vi "Module - Page Execute.vi"(11 "Stop":bool) -> ()   [LabVIEW 2020]
uses:
  Control/State - eFGV.ctl
  Control/Page - Execute State.ctl
  <vilib>/Utility/miscctls.llb/LVPointDoubleTypeDef.ctl
  Control/Section.ctl
  Control/Execute - Index of Elapse time.ctl
  Control/State - FGV.ctl
  <vilib>/Utility/NIReport.llb/NI_report.lvclass
  <vilib>/Utility/NIReport.llb/Report Type.ctl
  <vilib>/Utility/NIReport.llb/NI_ReportGenerationCore.lvlib
  Control/Setup - Sequence Data.ctl
  Control/Transaction Info.ctl
  Control/Product Info.ctl
  Control/Acceptance Criteria Info.ctl
  Control/Execution Info.ctl
  Control/Results Info.ctl
  Control/Data to Execute.ctl
  <vilib>/Utility/file.llb/Write Delimited Spreadsheet (string).vi
  <userlib>/_OpenG.lib/comparison/comparison.llb/Boolean Changed__ogtk.vi
  Control/Drop Rate Param.ctl
  Control/Control 1.ctl
  <vilib>/Utility/NIReport.llb/Append Report Text (str wrap).vi
  Control/Setup - Sequence Data Label.ctl
panel:
  out "String.Stabilizing status":string
  in  "End Mark":bool caption="1"
  out "Test Status Ind":string="Testing"
  out "SequenceNoFolder":string="SeqNo2"
  out "Hold Time Remainder":dbl=833.0095882415771
  in  "TARE":bool caption="1"
  in  "Test Type":string(combo)
  in  "Execute Tab":enum32{"Test", "Info", "Misc."}(tab)
  in  "Chart No":string
  in  "View":string(combo)="Polar Plot"
  in  "Test Category":string
  in  "TabControl.TestType":enum32{"Holding", "Blowdown"}(tab)
  out "%Pressure Stabilized":dbl caption="% of Current Pressure on Top of\nThe Test Pressure" format="%.1f"
  out "% Test Completed":dbl format="%.1f"
  out "Holding Started":bool
  out "Bool. Press Drop In Range":bool caption="Drop Rate Within Range"
  out "Pressure in Range":bool
  out "NumInd.BD_Pressure":sgl caption="Blowdown pressure (psi)" format="%.1f"
  out "Bool.BDTrig":bool caption="Blowdown Triggered"
  out "NumInd.2nd_pump_press":sgl caption="Second pump pressure (psi)" format="%.1f"
  out "Overall Status":bool
  in  "Table Reading":i32(listbox)
  out "Low Pressure":bool
  in  "Pause/Resume":bool
  in  "Execute View":string="View"
  in  "Execute Reading":string="Reading"
  in  "Execute Key Value":string="Key Value" caption="Info"
  in  "Execute Info":string="Info" caption="Info"
  out "Blow Down  Test":bool
  out "Hold Time (hh:mm)":string="00:15"
  out "Test Pressure":i32=15000 format="%.0f psi"
  in  "tab - View Data":T1(tab)
  in  "Start Marker":u32(colorbox)=16860
  in  "Plot Colour":u32(colorbox)=16711680
  in  "Stop Marker":u32(colorbox)=1441830
  in  "Grid Colour":u32(colorbox)=35170
  out "Polar Plot":picture
  out "Linear Graph":cluster{"Time ,x":dbl[], "Magnitude ,y":sgl[]}(graph)={"Time ,x"=[0.0, 0.9682250022888184, 1.9675369262695312, 2.9678306579589844, 3.9680562019348145, 4.9682745933532715, 5.967533111572266, 6.9688215255737305, 7.969114303588867, 8.969351291656494, 9.968575954437256, 10.968814373016357, 11.96904182434082, 12.96934986114502, 13.968584060668945, 14.968928813934326, 15.970189094543457, 16.969515323638916, 17.969897747039795, 18.970128059387207, 19.971360206604004, 20.97115707397461, 21.97089910507202, 22.971266269683838, 23.970398426055908, 24.970824718475342, 25.97111749649048, 26.97133207321167, 27.970609664916992, 28.97120952606201, 29.971484184265137, 30.971708297729492, 31.971967220306396, 32.97223615646362, 33.97146987915039, 34.97170972824097, 35.972264766693115, 36.9714994430542, 37.9732346534729, 38.97247362136841, 39.973758697509766, 40.973976135253906, 41.97420263290405, 42.97359752655029, 43.973846435546875, 44.97406625747681, 45.9743447303772, 46.97364091873169, 47.97390556335449, 48.9737114906311, 49.97393465042114, 50.973427295684814, 51.97372102737427, 52.974024295806885, 53.97428226470947, 54.97451066970825, 55.974753856658936, 56.975521087646484, 57.97573757171631, 58.97601938247681, 59.977320194244385, 60.97653150558472, 61.97792720794678, 62.97848987579346, 63.9788384437561, 64.97906398773193, 65.97934484481812, 66.97858905792236, 67.97981309890747, 68.98035621643066, 69.97958898544312, 70.98087692260742, 71.98110103607178, 72.98132658004761, 73.98166465759277, 74.98196268081665, 75.98217439651489, 76.98144865036011, 77.98171186447144, 78.98278427124023, 79.98302412033081, 80.98324394226074, 81.98297834396362, 82.98421907424927, 83.98345279693604], "Magnitude ,y"=[15033.86, 15033.86, 15033.86, 15033.86, 15033.86, 15033.86, 15033.86, 15033.86, 15033.86, 15033.86, 15033.86, 15033.86, 15033.86, 6252.822, 6252.822, 6252.822, 6252.822, 15011.287, 15011.287, 15011.287, 15011.287, 15011.287, 15011.287, 15011.287, 15011.287, 15011.287, 15011.287, 15011.287, 15011.287, 15011.287, 15011.287, 15011.287, 15011.287, 15011.287, 15011.287, 15011.287, 15011.287, 15011.287, 15011.287, 15011.287, 15011.287, 15011.287, 15011.287, 15011.287, 15011.287, 15011.287, 15011.287, 15011.287, 15011.287, 15011.287, 15011.287, 15011.287, 15011.287, 15011.287, 15011.287, 15011.287, 15011.287, 15011.287, 15011.287, 15011.287, 15011.287, 15011.287, 15011.287, 15011.287, 15011.287, 15011.287, 15011.287, 15011.287, 15011.287, 15011.287, 15011.287, 15011.287, 15011.287, 15011.287, 15011.287, 15011.287, 15011.287, 15011.287, 15011.287, 15011.287, 15011.287, 15011.287, 15011.287, 15011.287, 15011.287]}
  in  "Statistic":i32(listbox)
  out "Key Value Remain Hold Time":string="00:00:00" caption="Holding Time Duration"
  out "Key Value Recording Duration":string="00:01:24" caption="Recording Duration"
  out "Key Value Current Pressure (psi)":sgl=15011.287 caption="Current Pressure (psi)"
  in  "Start Test":bool caption="1"
  out "Remaining Hold Time":string="00:00:00"
  out "Holding Pressure (psi)":dbl=15000.0
  out "Current Pressure (psi)":sgl
  in  "Clear Mark":bool caption="1"
  in  "Start Mark":bool caption="1"
  in  "Finish":bool caption="1"
  out "Start Holding Datetime":string="22.June.2022 06:14:10"
  out "Recorded Holding Time":string="00:03:00"
  out "Start Holding Pressure (psi)":string="15011.3"
  out "Different in Holding Pressure,psi(%)":string="0.0 psi(0.0 %)"
  out "Permitted Holding Pressure Drop, psi%":string="450.0 psi(3.0 %)"
  out "Recording Duration":string="00:00:00"
  out "Test Sequence":string="5"
  out "Seq.No":string="2"
  out "Variance":string="All"
  out "Transaction Number":u16=3
  out "Test Requirement":string="Hydro Open Body Test"
  out "Test Media":string="Water"
  out "Indicator.PressureDropRatePsi":dbl caption="Pressure Drop Rate" format="%.1f psi/hr"
  out "Indicator.PressureDropRate%":dbl caption="Pressure Drop Rate(psi/hr)" format="%.1f %%"
  out "Notes":string
  out "PSL":string
  in  "Test System Description":string caption="Test System"
  out "Rework":bool caption="Rework?"
  out "Ref Order No.":dbl caption="Ref. Order No."
  out "NCR No.":string
  in  "Header multi-test 3":T2={"Seq.Done"="Status", "Label.RunSeq"="Select", "Label.TestSeq"="Run?", "Label.SeqNo"="Test Sequence", "Seq.No 4"="Test Req. ID", "Seq.No 5"="Test Requirement", "Seq.No 6"="Variance", "Seq.No 7"="Test Procedure", "Seq.No 8"="Section", "Seq.No 9"="Test Bunker", "Seq.No 10"="Test Media", "Seq.No 11"="Test Pressure (psi)", "Seq.No 12"="Cycle", "Seq.No 13"="Holding time (hh:mm)", "Seq.No 14"="Chart Scale", "Seq.No 15"="Blowdown? (y/n)", "Seq.No 16"="Actuator Pressure (psi)", "Seq.No 17"="Max. Blowdown Pressure (psi)", "Label.SelectSeq"="No.", "Bool.SelectSeq"=FALSE, "Bool.RunSeq"=FALSE, "Bool.TestSeq"=FALSE, "Bool.SeqNo"=FALSE, "Label.TestGroup"="Test Group", "Bool.TestGroup"=FALSE, "Seq.MSHP"="MSHP", "Seq.PHPD"="PHPD"}
  out "Sequence List":T3[](array[typedef])=[{"Seq.Select"=FALSE, "Seq.Status"=6618880, "Seq.Run"=TRUE, "Seq.TestSequence"="5", "Seq.No"="1", "Seq.ReqID"="", "Seq.TestReq"="Hydro Open Body Test", "Seq.Variance"="All", "Seq.TestProcedure"="X-???", "Seq.Section"="???", "Seq.TestBunker"="SB SUT 1", "Seq.TestMedia"="Water", "Seq.TestPressure"="15000", "Seq.Cycle"="Primary", "Seq.HoldingTime"="00:03", "Seq.ChartScale"="", "Seq.BDIndicator"="N", "Seq.ActuatorPressure"="", "Seq.MaxBDPressure"=""}, {"Seq.Select"=FALSE, "Seq.Status"=3381759, "Seq.Run"=TRUE, "Seq.TestSequence"="5", "Seq.No"="2", "Seq.ReqID"="", "Seq.TestReq"="Hydro Open Body Test", "Seq.Variance"="All", "Seq.TestProcedure"="X-???", "Seq.Section"="???", "Seq.TestBunker"="SB SUT 1", "Seq.TestMedia"="Water", "Seq.TestPressure"="15000", "Seq.Cycle"="Secondary", "Seq.HoldingTime"="00:15", "Seq.ChartScale"="", "Seq.BDIndicator"="N", "Seq.ActuatorPressure"="", "Seq.MaxBDPressure"=""}, {"Seq.Select"=FALSE, "Seq.Status"=16711680, "Seq.Run"=TRUE, "Seq.TestSequence"="6", "Seq.No"="3", "Seq.ReqID"="", "Seq.TestReq"="Hydraulic Actuator/Bonnet Interface (PMV)", "Seq.Variance"="PMV", "Seq.TestProcedure"="X-341926-01", "Seq.Section"="???", "Seq.TestBunker"="SB SUT 1", "Seq.TestMedia"="Control Fluid", "Seq.TestPressure"="100", "Seq.Cycle"="Single Cycle", "Seq.HoldingTime"="00:03", "Seq.ChartScale"="", "Seq.BDIndicator"="N", "Seq.ActuatorPressure"="", "Seq.MaxBDPressure"=""}, {"Seq.Select"=FALSE, "Seq.Status"=16711680, "Seq.Run"=TRUE, "Seq.TestSequence"="6", "Seq.No"="4", "Seq.ReqID"="", "Seq.TestReq"="Hydraulic Actuator/Bonnet Interface (AMV)", "Seq.Variance"="AMV", "Seq.TestProcedure"="X-341926-01", "Seq.Section"="???", "Seq.TestBunker"="SB SUT 1", "Seq.TestMedia"="Control Fluid", "Seq.TestPressure"="100", "Seq.Cycle"="Single Cycle", "Seq.HoldingTime"="00:03", "Seq.ChartScale"="", "Seq.BDIndicator"="N", "Seq.ActuatorPressure"="", "Seq.MaxBDPressure"=""}]
  in  "Label.Test":string="Test" caption="Test"
  out "Test Category list":string="SUT 9, Hydro"
  in  "Test System":string
  in  "Test Category":string
  out "Material Description":string caption="Material List"
  out "Material":string="0"
  out "Project":string
  out "Customer Description":string caption="Customer List"
  in  "Test System Name":string
  in  "Procedure No./Ref.":string="X2345.xlsx" caption="X-Document No./Ref."
  out "Working Pressure":string
  in  "Test System":string
  out "Rev.":string
  out "Product Category":string
  out "BOM Rev.":dbl
  out "Sale Order":string="0" caption="Sales Order"
  out "Customer":string="0"
  out "NCR":string
  out "Order Number":string="0"
  out "Quantity":u16=1 min=1 step=1
  in  "Default View":string(combo)="Polar Plot"
  in  "View Change Duration":dbl=1.0 caption="Return to default view after" min=0.1 max=60.0 step=0.1 format="%.1f minutes"
  in  "Label.View change":string="Production Order Details" caption="Production Order Details"
  out "Enum.Pressure stabilize wait time":enum16{"seconds", "minutes"}(ring)=enum."minutes"
  out "Pressure stabilize wait time":dbl=10.0 min=0.0 max=100.0
  out "Auto Stop Test":bool caption="Automatic Stop Test after Hold Time Countdown"
  out "Auto Set Marker":bool=TRUE caption="Automatic set start marker upon pressure stabilized"
  in  "Header.Tool":T4={"Type "="Type", "Id"=" ID", "Description"="Description", "Serial No"="Serial No"} caption="Header Tool"
  out "Table.Tool":i32(listbox) caption="Detail Sensor"
  out "Table.Sensor":i32(listbox) caption="Detail Sensor"
  in  "Header.Sensor":T5={"Type "="Type", "Id"=" ID", "Description"="Description", "Serial No"="Serial No", "LP"="LP"} caption="Header Detail Sensor"
  in  "Label.Result":string="Result" caption="Result"
  out "Output Set Company":string
  out "ListBox.Output Set":string="1001.xltx" caption="Output Set"
  in  "Label.Production Order Details":string="Production Order Details" caption="Production Order Details"
  out "Indicator.Sub Operation":string caption="Sub Operation"
  out "Indicator.Confirmation No":u32 caption="Confirmation No"
  out "Indicator.Operation":string caption="Operation"
  out "Indicator.Sequence No":u16 caption="Sequence No"
  out "Indicator.Order Number":u32 caption="Order Number"
  in  "Label.Tools":string="Tools" caption="Tools"
  in  "Label.Sensor":string="Sensor" caption="Sensor"
  in  "Label.Additional Procedures No./Ref.":string="Additional Procedures No./Ref." caption="Additional Procedures No./Ref."
  out "Table.Procedure No./Ref.":i32(listbox)
  out "Acceptance Criteria":string="Acceptance Criteria"
  out "% Permitted Holding Pressure":string="% per hour (vs. start holding pressure)"
  out "% Test Pressure":string="% on top of the test pressure"
  out "Permitted Holding Pressure Drop":dbl=3.0
  out "Max Start Holding Pressure":dbl=3.0 caption="Maximum Start Of Holding Pressure"
  # "EXECUTE"
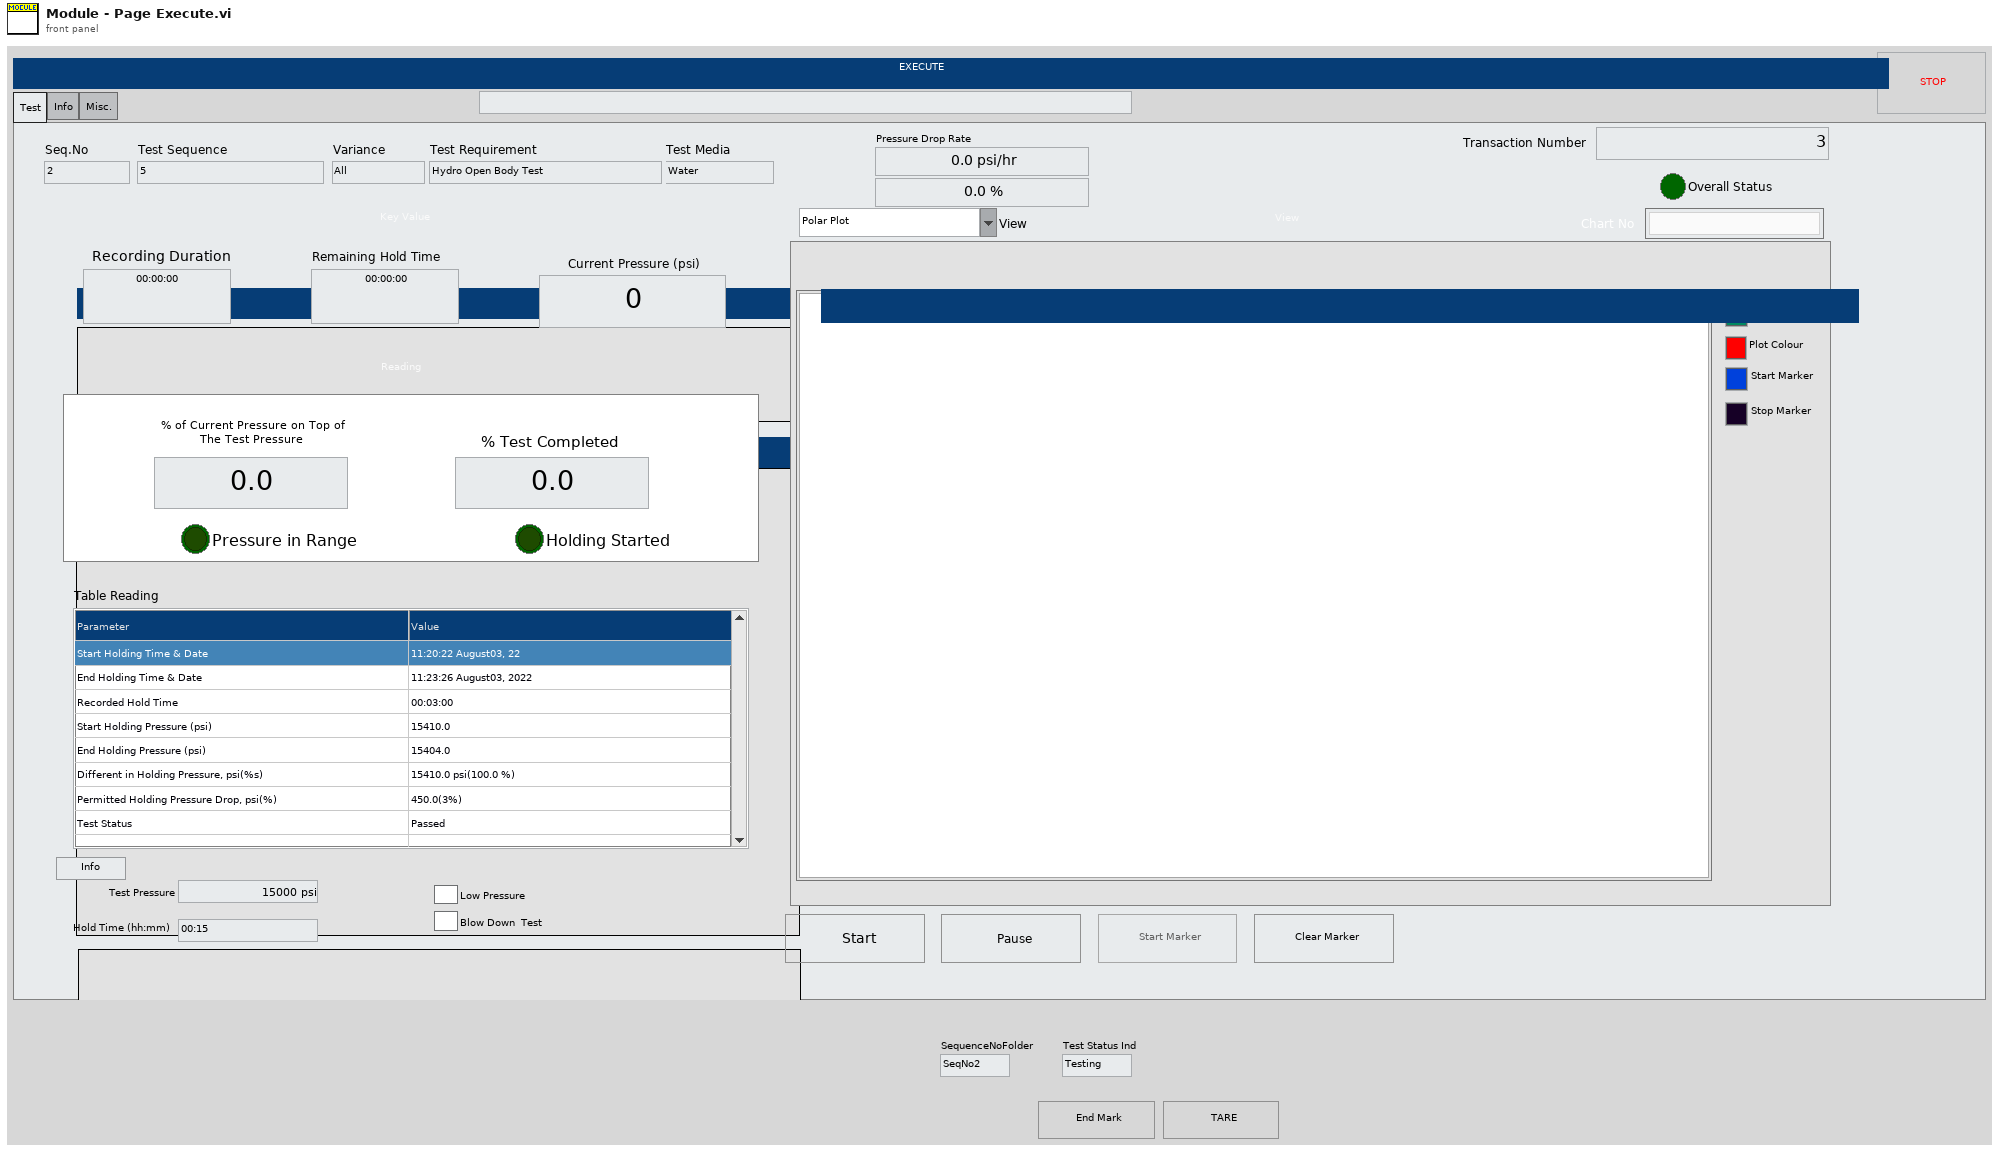
[diagram p1: front panel]
types:
  T1 = enum32{"Polar Plot", "Linear", "Statistic", "Key Value"}
  T2 = typedef "Setup - Sequence Data Label.ctl" = cluster{"Seq.Done":string, "Label.RunSeq":string, "Label.TestSeq":string, "Label.SeqNo":string, "Seq.No 4":string, "Seq.No 5":string, "Seq.No 6":string, "Seq.No 7":string, "Seq.No 8":string, "Seq.No 9":string, "Seq.No 10":string, "Seq.No 11":string, "Seq.No 12":string, "Seq.No 13":string, "Seq.No 14":string, "Seq.No 15":string, "Seq.No 16":string, "Seq.No 17":string, "Label.SelectSeq":string, "Bool.SelectSeq":bool, "Bool.RunSeq":bool, "Bool.TestSeq":bool, "Bool.SeqNo":bool, "Label.TestGroup":string, "Bool.TestGroup":bool, "Seq.MSHP":string, "Seq.PHPD":string}
  T3 = typedef "Setup - Sequence Data.ctl" = cluster{"Seq.Select":bool, "Seq.Status":u32, "Seq.Run":bool, "Seq.TestSequence":string, "Seq.No":string, "Seq.ReqID":string, "Seq.TestReq":string, "Seq.Variance":string, "Seq.TestProcedure":string, "Seq.Section":string, "Seq.TestBunker":string, "Seq.TestMedia":string, "Seq.TestPressure":string, "Seq.Cycle":string, "Seq.HoldingTime":string, "Seq.ChartScale":string, "Seq.BDIndicator":string, "Seq.ActuatorPressure":string, "Seq.MaxBDPressure":string}
  T4 = cluster{"Type ":string, "Id":string, "Description":string, "Serial No":string}
  T5 = cluster{"Type ":string, "Id":string, "Description":string, "Serial No":string, "LP":string}
  T6 = typedef "Execute - Index of Elapse time.ctl" = enum16{"Elapse Gap Data", "Holding Time", "Recording Duration", "View Change", "Pressure stabilize timer", "Press. Drop Rate", "Init Holding Buffer"}
  T7 = typedef "Data to Execute.ctl" = cluster{"Transaction Info":T8, "Product Info":T9, "Misc - Additional Refs":string[][], "Misc - Sensors":string[][], "Misc - Tools":string[][], "Acceptance Criteria Info":T10, "Execution Info":T11, "Results Info":T12, "Notes":string}
  T8 = typedef "Transaction Info.ctl" = cluster{"Transaction Number":string, "Order Number":string, "Quantity":u16, "Customer":u32, "Customer Description":string, "Project":string, "Sales Order":u32, "Material":string, "Material Description":string, "Rework":bool, "NCR No.":string, "Ref Order No.":string, "Item No.":u32, "BOM Rev.":dbl}
  T9 = typedef "Product Info.ctl" = cluster{"Product Category":string, "Procedure No./Ref.":string, "Test System":string, "Test System Description":string, "Working Pressure":string, "Pressure Unit":string, "Rev.":string, "PSL":string}
  T10 = typedef "Acceptance Criteria Info.ctl" = cluster{"Max Start Hold Pressure":dbl, "Enum.Max Start Hold Pressure":enum16{"%", "psi"}, "Permitted Hold Pressure Drop":dbl, "Enum.Permitted Hold Pressure Drop":enum16{"%", "psi"}, "Pressure stabilize wait time":dbl, "Enum.Pressure stabilize wait time":enum16{"seconds", "minutes"}}
  T11 = typedef "Execution Info.ctl" = cluster{"Auto Set Marker":bool, "Auto Stop Test":bool}
  T12 = typedef "Results Info.ctl" = cluster{"ListBox.Output Set":string, "Output Set Description":string}
  T13 = typedef "Setup - Sequence Data.ctl" = cluster{"Seq.Select":bool, "Seq.Status":u32, "Seq.Run":bool, "Seq.TestSequence":dbl, "Seq.No":dbl, "Seq.ReqID":string, "Seq.TestReq":string, "Seq.Variance":string, "Seq.TestProcedure":string, "Seq.Section":string, "Seq.TestSystem":string, "Seq.TestPressure":string, "Seq.Cycle":string, "Seq.TestGroup":dbl, "Seq.MSHP":dbl, "Seq.PHPD":dbl, "Seq.HoldingTime":string, "Seq.ChartScale":string, "Seq.ActuatorPressure":string, "Seq.MaxBDPressure":string, "Seq.BDIndicator":bool, "Seq.TestMedia":string}
  T14 = typedef "Drop Rate Param.ctl" = cluster{"Drop Rate Calc Interval (sec)":dbl, "Last Pressure (psi)":dbl, "Allowable Press. Drop/min":dbl, "Pressure Drop Accepted?":bool, "Block interval to test":i32, "Block counter":i32, "Allowable Press. Drop/hr":dbl}
  T15 = typedef "Control 1.ctl" = enum32{"Holding", "Blowdown"}
  T16 = cluster{"T_Out":i32, "Point Phase":dbl[], "polar attributes":cluster{"maximum":dbl, "minimum":dbl, "clip to min":bool, "log?(F)":bool, "grid color":u32, "plot color":u32, "fmt and prec":cluster{"format":enum8{"Decimal", "Scientific", "Engineering", "Binary", "Octal", "Hex"}, "precision":u8}, "visible section":u16}, "Current Pressure":sgl, "Counter Time":dbl, "marking plot colour":u32, "Active Cursor":u32, "Event AI Data":sgl[], "Run Test":bool, "Config":cluster{"Holding Pressure":dbl, "Set Polar Time":dbl}, "Array of Elapse Time":timestamp[], "Remaining Holding Time":dbl, "Max Pressure":sgl, "Start Mark":bool, "Plot length (min)":dbl, "Plot length scale":dbl, "Magnitude ,y":sgl[], "Time ,x":dbl[], "Result Elapse":dbl[], "Phase":dbl[], "data array [mag, phase (deg)]":cluster{"magnitude":dbl, "phase":dbl}[], "Max Phase":dbl, "Plot and scale":cluster{"Size Linear plot":u16, "Size point plot":u16, "Plot Scale":dbl}, "Start Holding Pressure (psi)":dbl, "End Holding Pressure (psi)":dbl, "Marking Data":cluster{"magnitude 2":dbl, "phase":dbl}[], "Display Polar Scale":cluster{"Time Scale Label":string, "Max Scale label":string}, "report out":refnum<class "NI_report.lvclass">, "axis labels":string[], "Polar Picture":picture, "Event Ref":refnum<event-registration>, "Data to Execute":T7, "Sequence Data":T13[], "Holding Started?":bool, "%Pressure Stabilized":dbl, "Target Holding Time":dbl, "Datalog path":path, "AI Offset":sgl[], "Sequence Number":i32, "Current Sequence":T13, "All Sequence Done":bool, "Sequence Started":bool, "Default View":string, "View Change Duration":dbl, "First data point?":bool, "Test Pressure Range":cluster{"Maximum":dbl, "Minimum":dbl, "Pressure in range?":bool}, "Stabilizing wait time":dbl, "Run Pressure Data":cluster{"Max Pressure":dbl, "Min Pressure":dbl, "Max Pressure TS":timestamp, "Min Pressure TS":timestamp}, "Drop Rate Param":T14, "TestType":T15, "Blowdown Param":cluster{"Actuator Pressure":dbl, "Max BD Pressure":dbl, "BD Triggered":bool, "BD Pressure":dbl}}
  T17 = typedef "Page - Execute State.ctl" = enum16{"Init", "Register Event", "Read Config File", "Idle", "Start Marking", "Clear Mark", "Init Test Param", "Init File and Folder", "Get Current Sequence", "Get pressure range", "Holding - Cal Elapse Time", "Get Current Pressure", "Calc. press. drop rate", "Check pressure in range", "Calc. stabilizing elapsed time", "Calc - Holding start Buffer Time", "Calc. Max Min Pressure", "Display Data", "Check Start Holding", "Blowdown - Check BD Trigger", "Blowdown - Mark BD", "Polar attributes", "Insert Acc Data", "Convert Time To Phase", "Get Plot length", "Polar linear Plot", "Polar Point", "Plot linear Graph", "Update Table Data", "Display Holding Time", "Display Result Test", "Display Label", "Finish Test", "Setup Cop", "Merge Picture", "Save  Data", "Get Next Sequence", "Create Report", "Fillup Report", "Process", "Update Info - Transaction", "Update Info - Product", "Update Info - Additional Refs", "Update Info - Sensors", "Update Info - Tools", "Update Info - Acceptance Criteria", "Update Info - Execution", "Update Info - Results", "Update Info - Notes", "Close"}
  T18 = typedef "Section.ctl" = enum16{"Software Setup", "Config", "Setup", "Network Stream", "MQTT Client", "Setting", "Sample Interval", "Calibration", "Pre-Ranging", "Overrun", "Static", "Filter", "Properties", "Alarm", "Device", "Logging"}
  T19 = typedef "LVPointDoubleTypeDef.ctl" = cluster{"X":dbl, "Y":dbl}
  T20 = typedef "State - FGV.ctl" = enum16{"Write", "Read"}
  T21 = enum8{"Decimal", "Scientific", "Engineering", "Binary", "Octal", "Hex"}
  T22 = cluster{"polar attributes":cluster{"maximum":dbl, "minimum":dbl, "clip to min":bool, "log?(F)":bool, "grid color":u32, "plot color":u32, "fmt and prec":cluster{"format":enum8{"Decimal", "Scientific", "Engineering", "Binary", "Octal", "Hex"}, "precision":u8}, "visible section":u16}, "data array [mag, phase (deg)]":cluster{"magnitude":dbl, "phase":dbl}[], "font":cluster{"desired font(Application) ":enum16{"User-specified Font", "Application Font", "System Font", "Dialog Font"}, "[user-specified font] ":cluster{"Font Name:":string, "Size":i16, "Strikeout?":bool, "Italic?":bool, "Underline?":bool, "Outline?":bool, "Shadow?":bool, "Bold?":bool}}, "Scale Polar plot":dbl, "Size":u16}
  T23 = cluster{"Execute Data":string[], "Sequence no":string}
  T24 = typedef "State - eFGV.ctl" = enum16{"Init", "Read", "Write", "Exit"}
  T25 = typedef "NI_ReportGenerationCore.lvlib/Report Type.ctl" = enum16{"HTML", "Word", "Excel"}
  T26 = cluster{"position (excel)":cluster{"row":i32, "column":i32}, "name (excel)":string, "bookmark (word)":string}
  T27 = enum8{"Enabled", "Disabled", "Disabled and Grayed Out"}
  T28 = cluster{"Maximum":dbl, "Minimum":dbl, "Pressure in range?":bool}
  T29 = cluster{"Size Linear plot":u16, "Size point plot":u16, "Plot Scale":dbl}
  T30 = cluster{"maximum":dbl, "minimum":dbl, "clip to min":bool, "log?(F)":bool, "grid color":u32, "plot color":u32, "fmt and prec":cluster{"format":enum8{"Decimal", "Scientific", "Engineering", "Binary", "Octal", "Hex"}, "precision":u8}, "visible section":u16}
  T31 = typedef "LVBoundsTypeDef.ctl" = cluster{"Width":u32, "Height":u32}
  T32 = typedef "imagedata.ctl" = cluster{"image type":i32, "image depth":i32, "image":u8[], "mask":u8[], "colors":u32[], "Rectangle":cluster{"left":i16, "top":i16, "right":i16, "bottom":i16}}
  T33 = enum32{"invalid app kind", "Development System", "Run Time System", "Student Edition", "Embedded LabVIEW", "Evaluation", "Custom"}
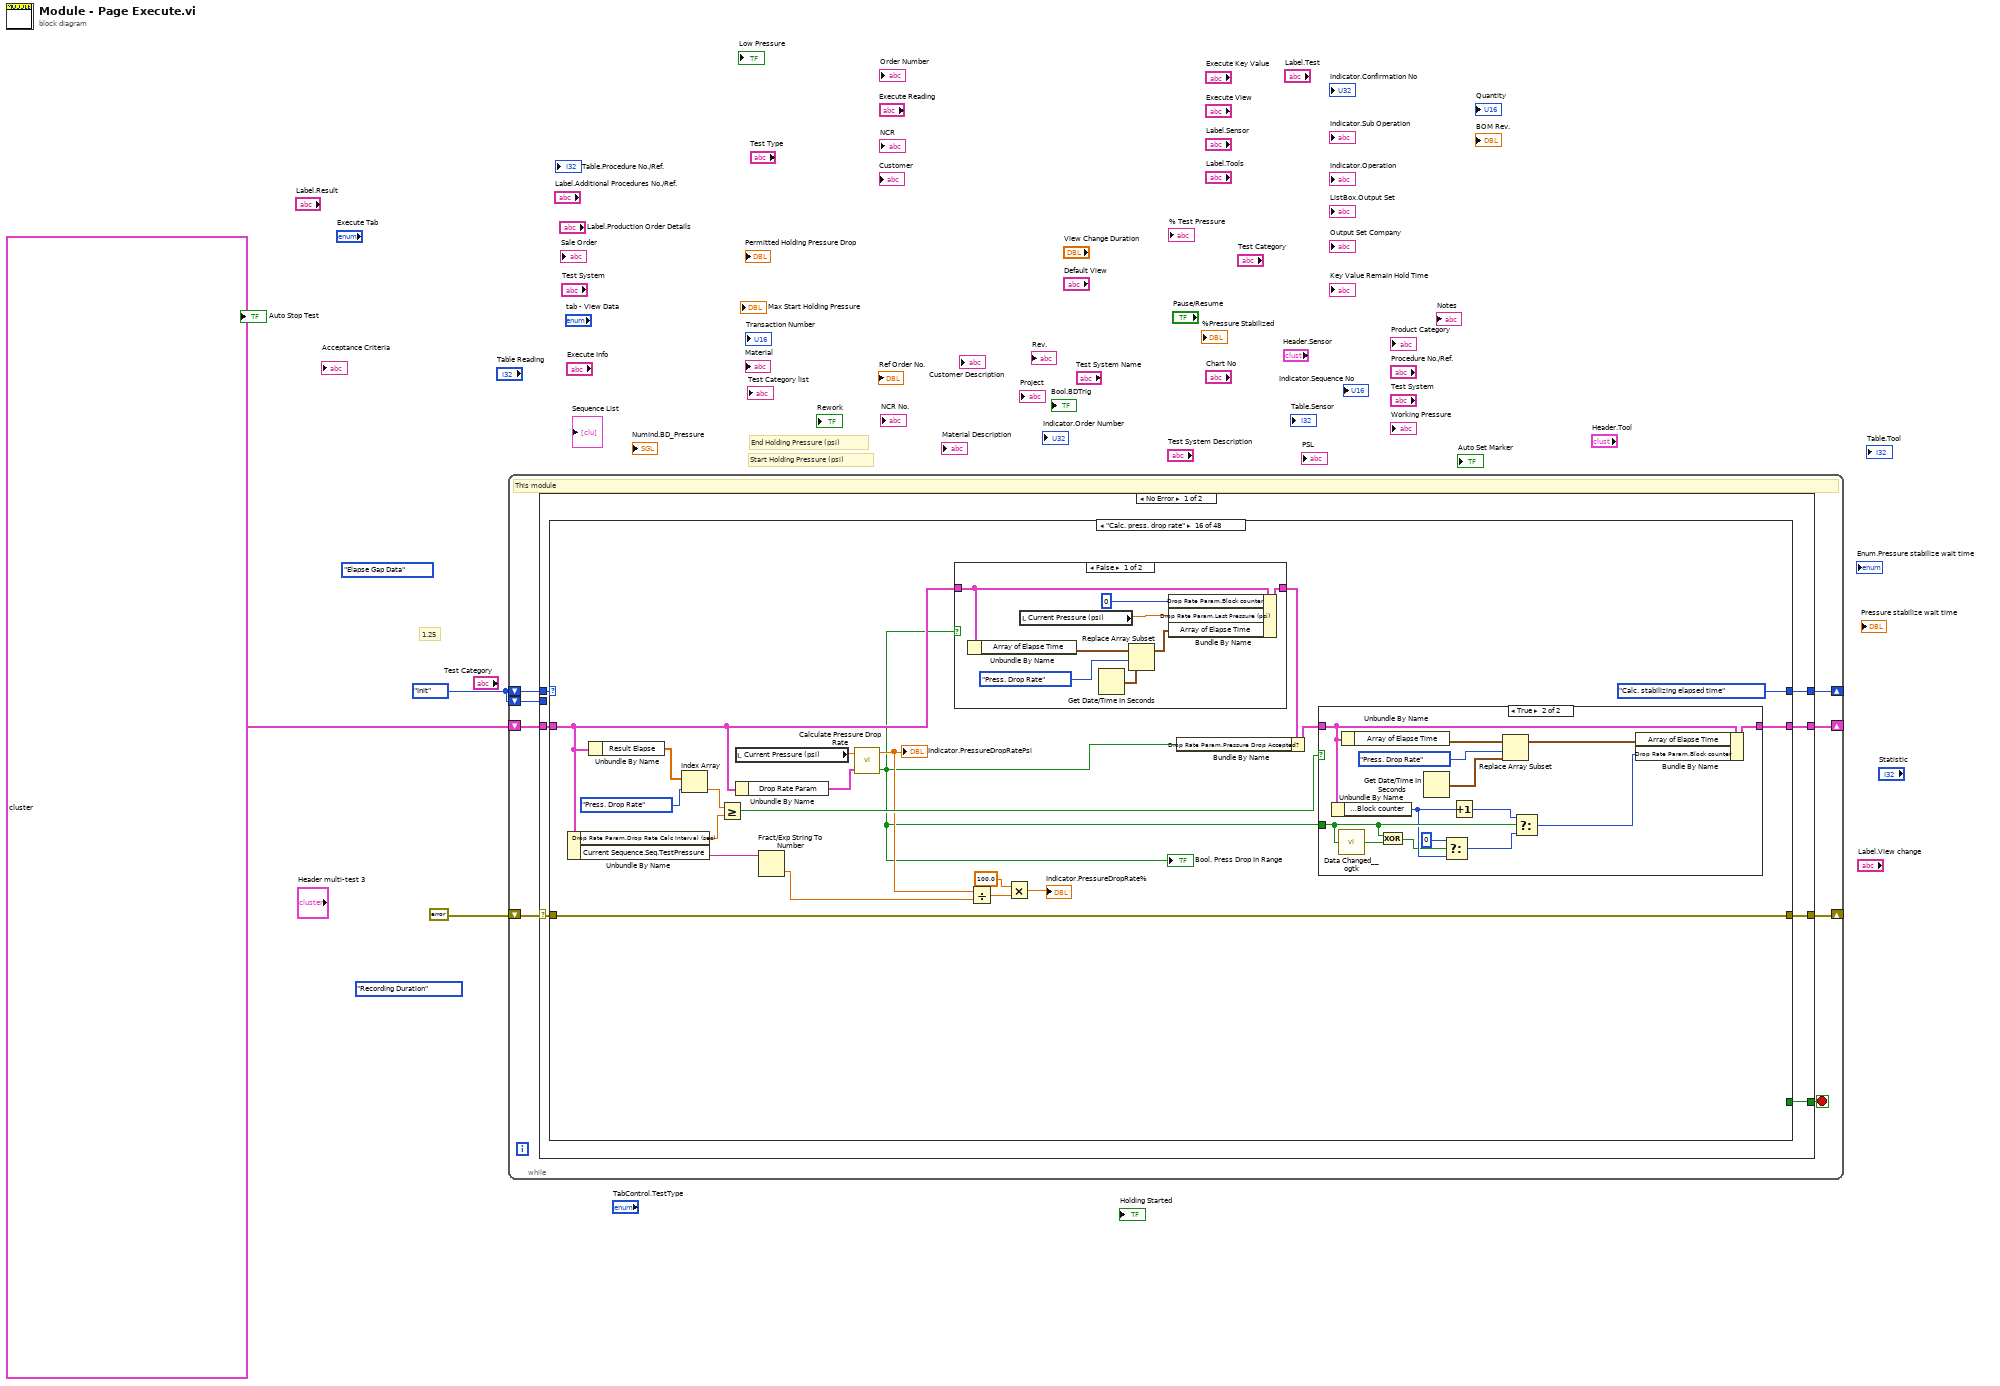
[diagram p0: block diagram]
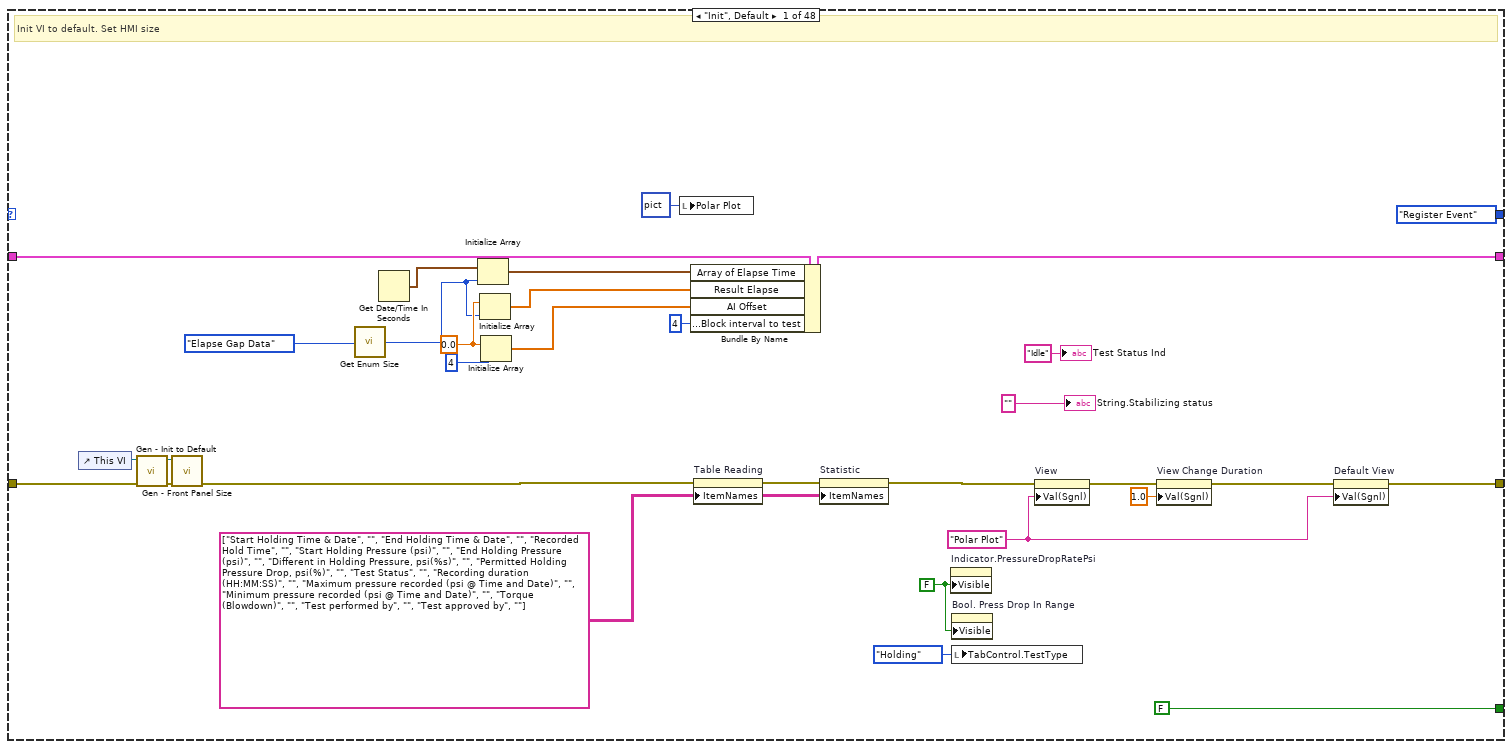
[diagram p2: hidden frame]
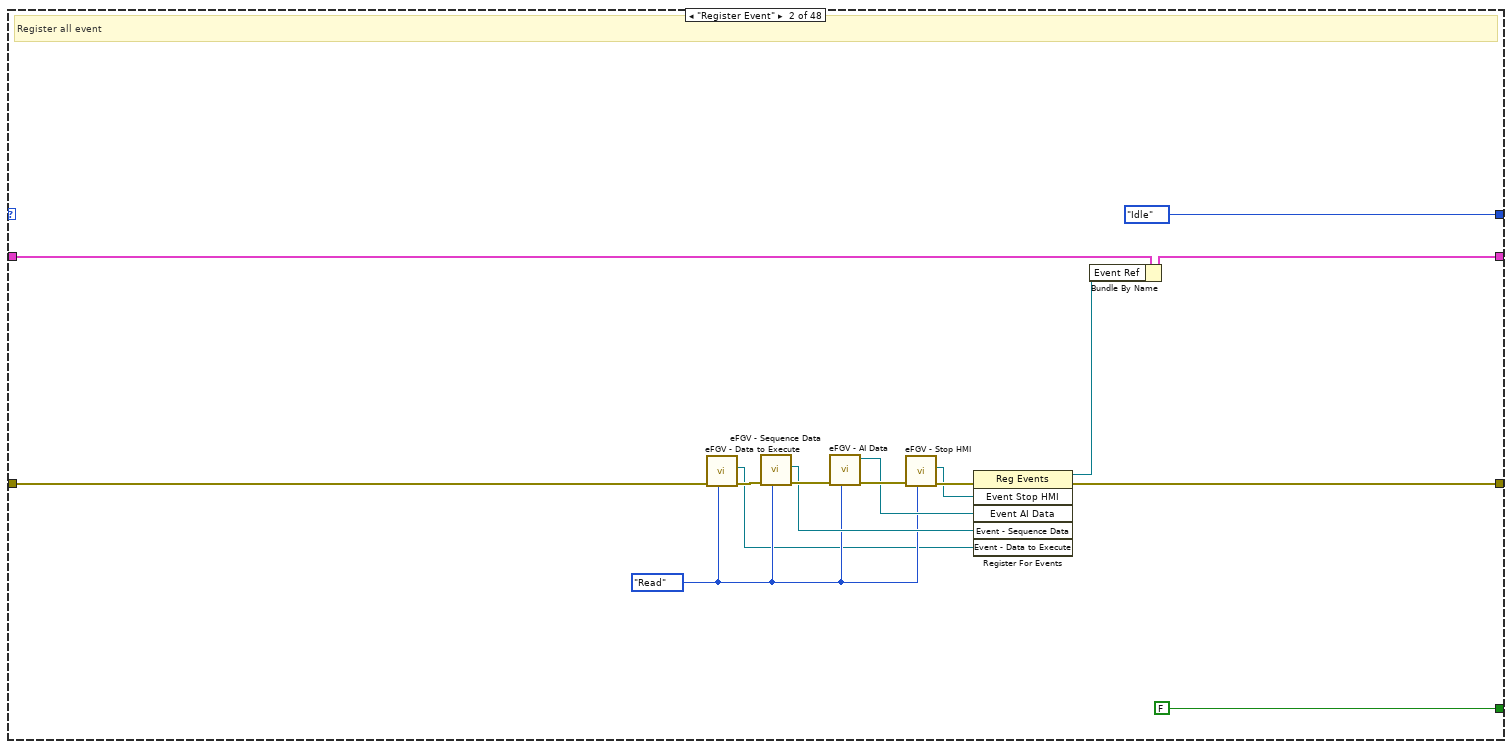
[diagram p3: hidden frame]
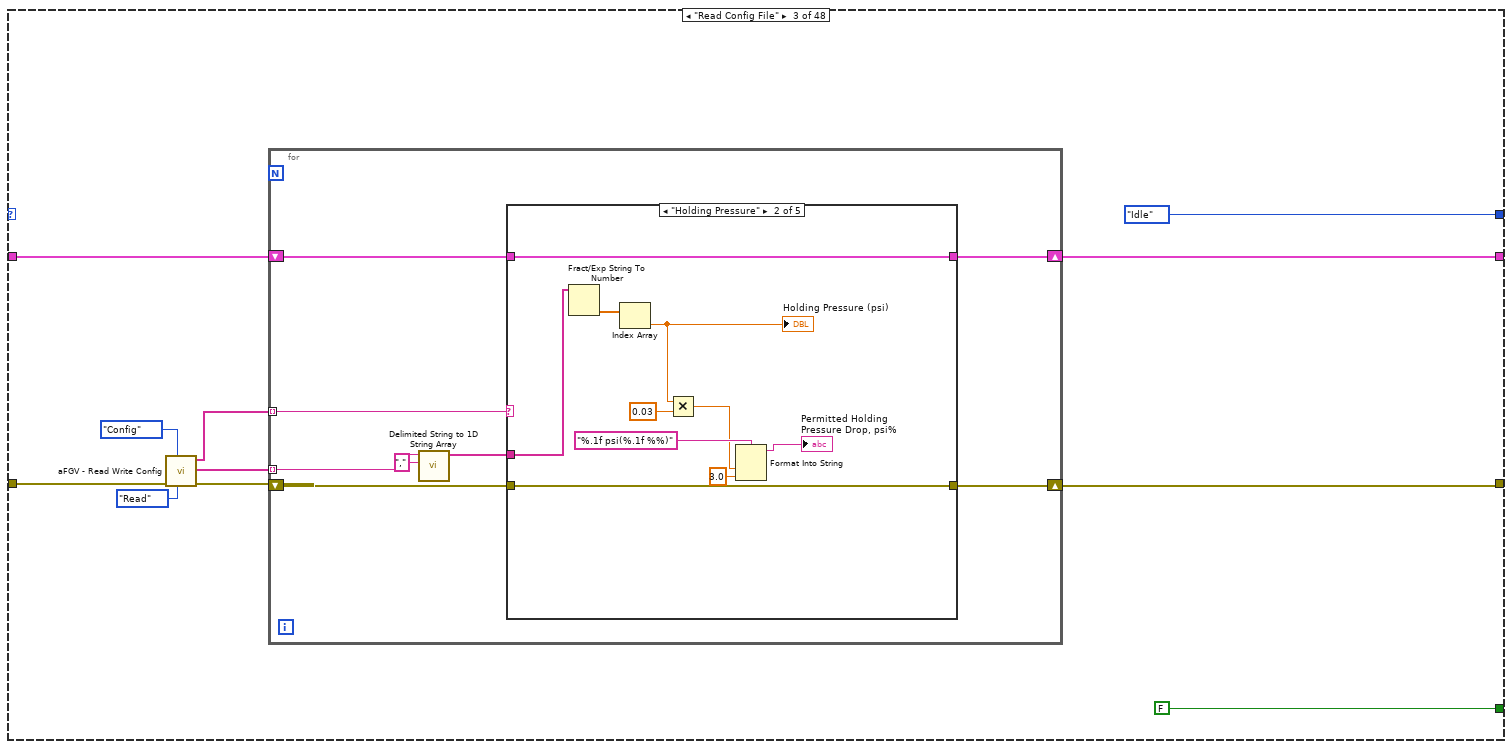
[diagram p4: hidden frame]
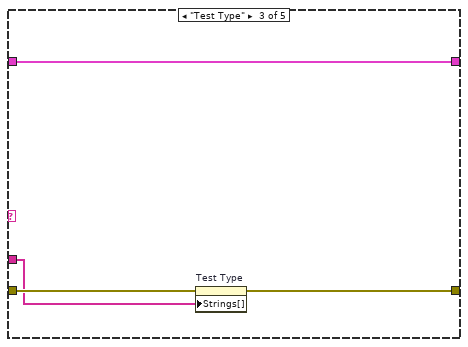
[diagram p6: hidden frame]
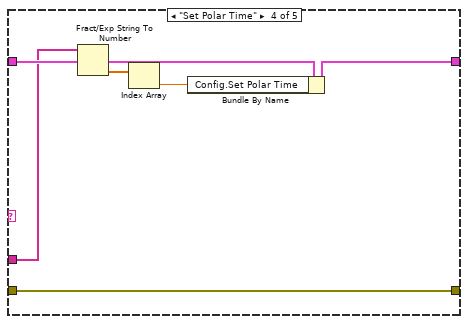
[diagram p7: hidden frame]
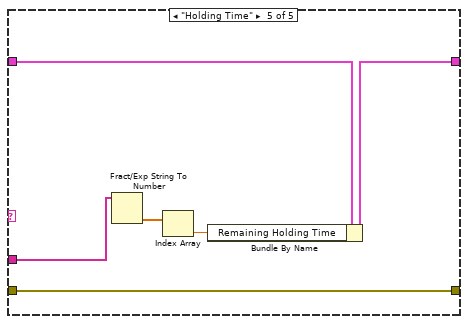
[diagram p8: hidden frame]
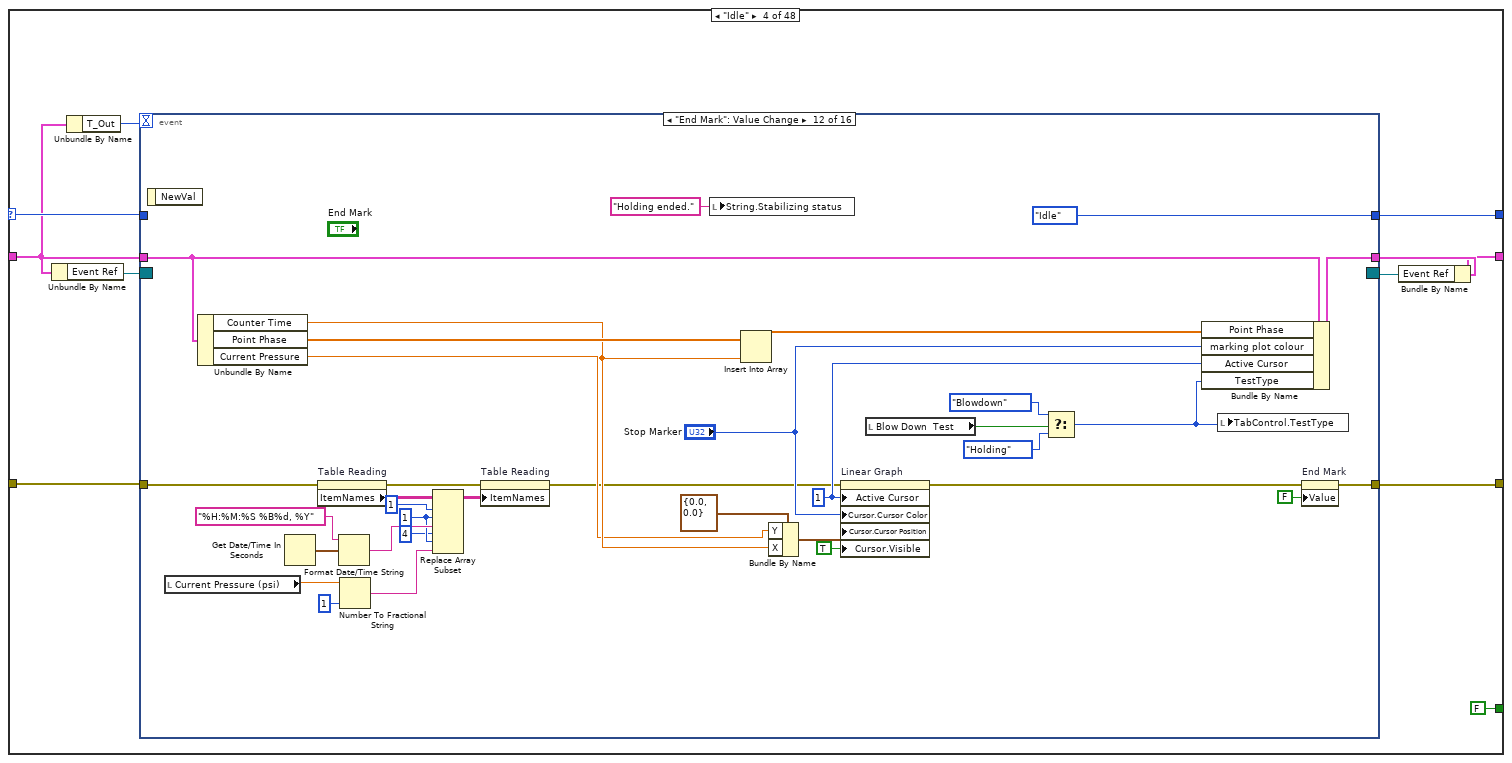
[diagram p9: hidden frame]
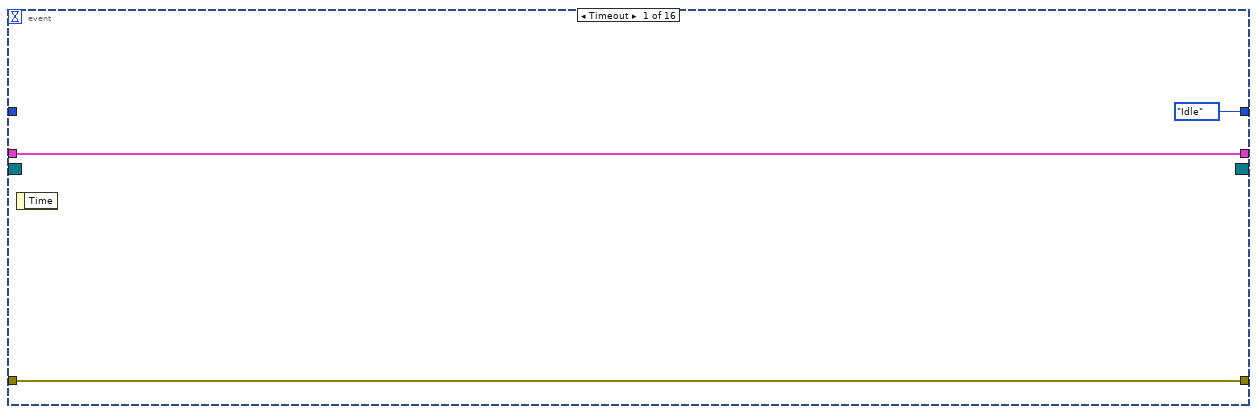
[diagram p10: hidden frame]
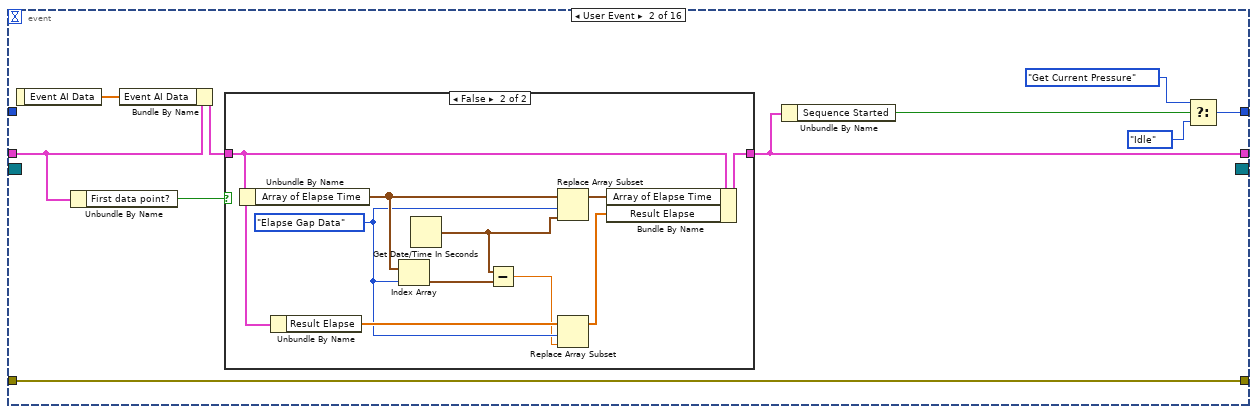
[diagram p11: hidden frame]
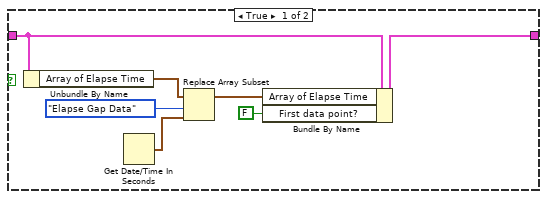
[diagram p12: hidden frame]
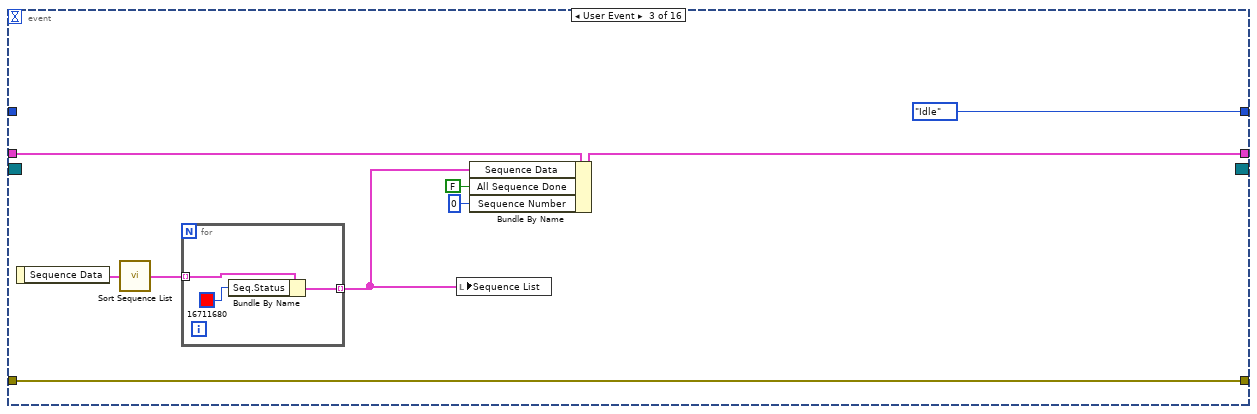
[diagram p13: hidden frame]
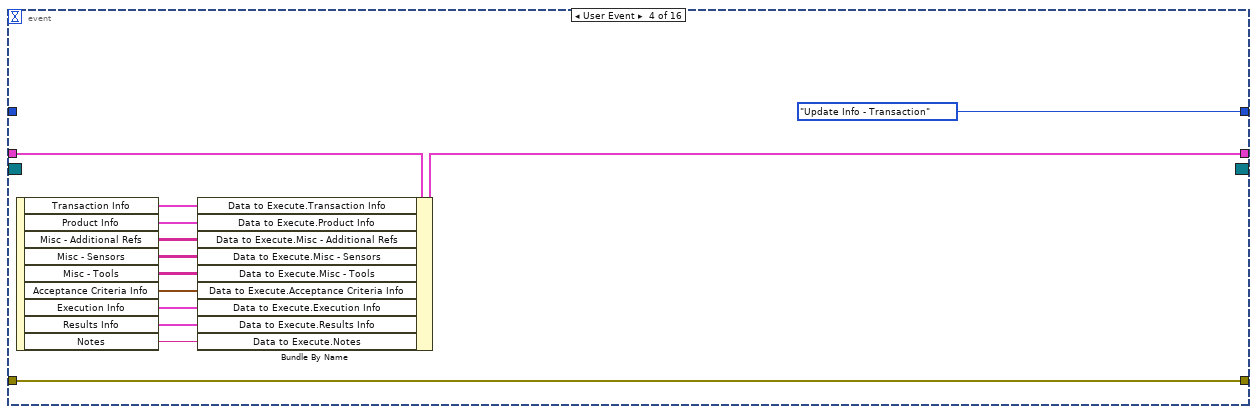
[diagram p14: hidden frame]
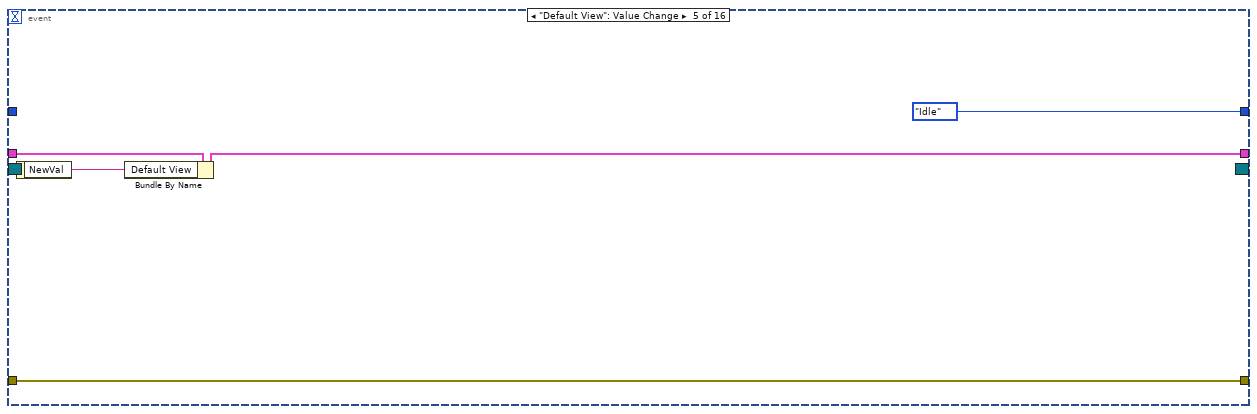
[diagram p15: hidden frame]
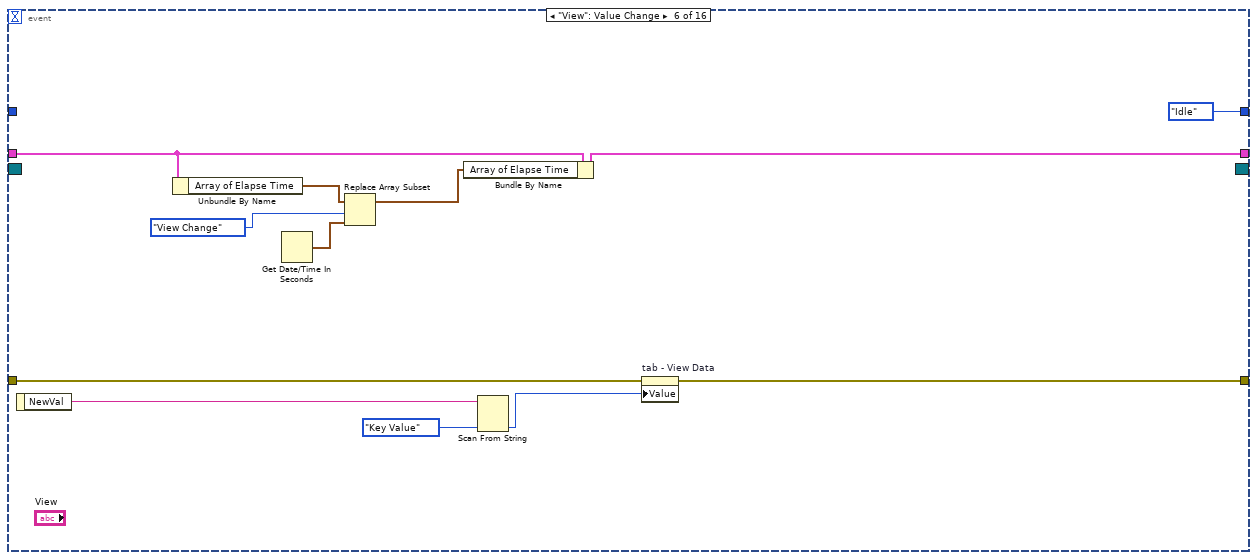
[diagram p16: hidden frame]
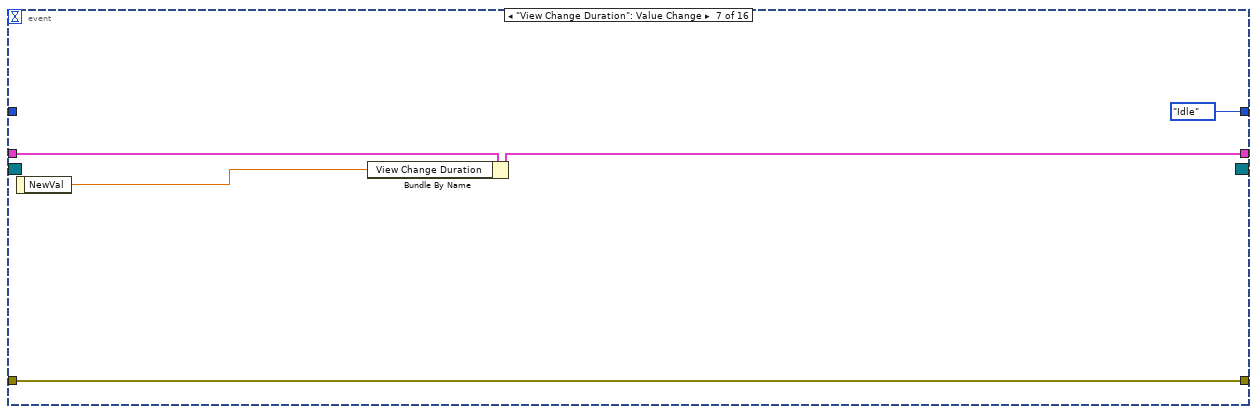
[diagram p17: hidden frame]
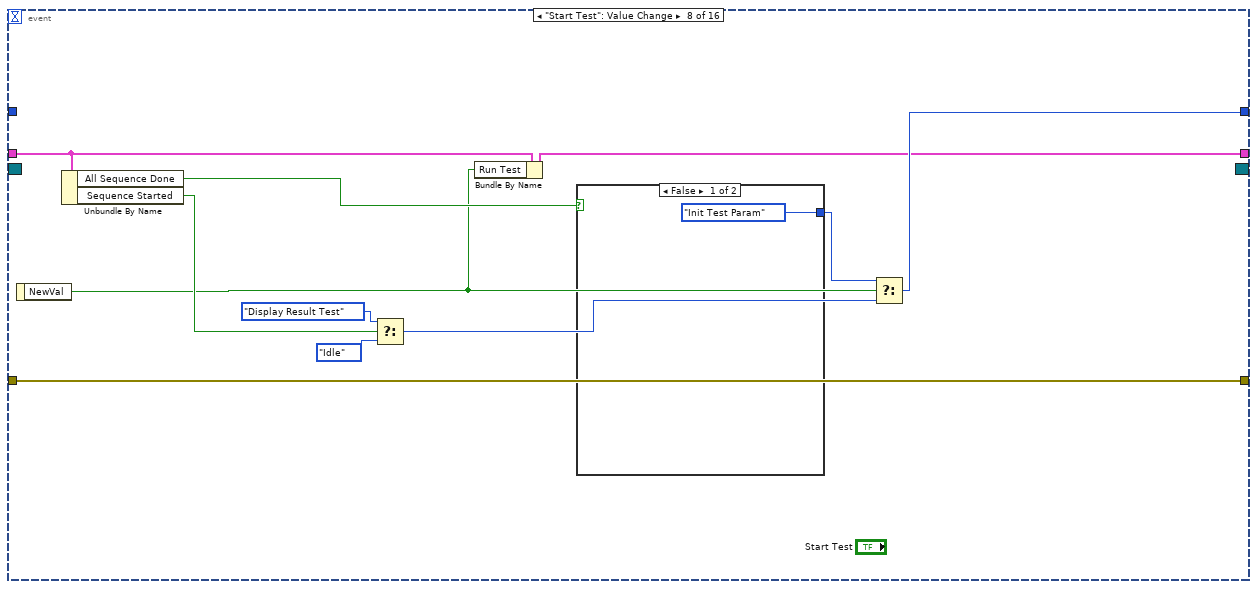
[diagram p18: hidden frame]
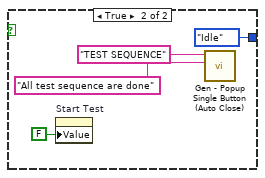
[diagram p19: hidden frame]
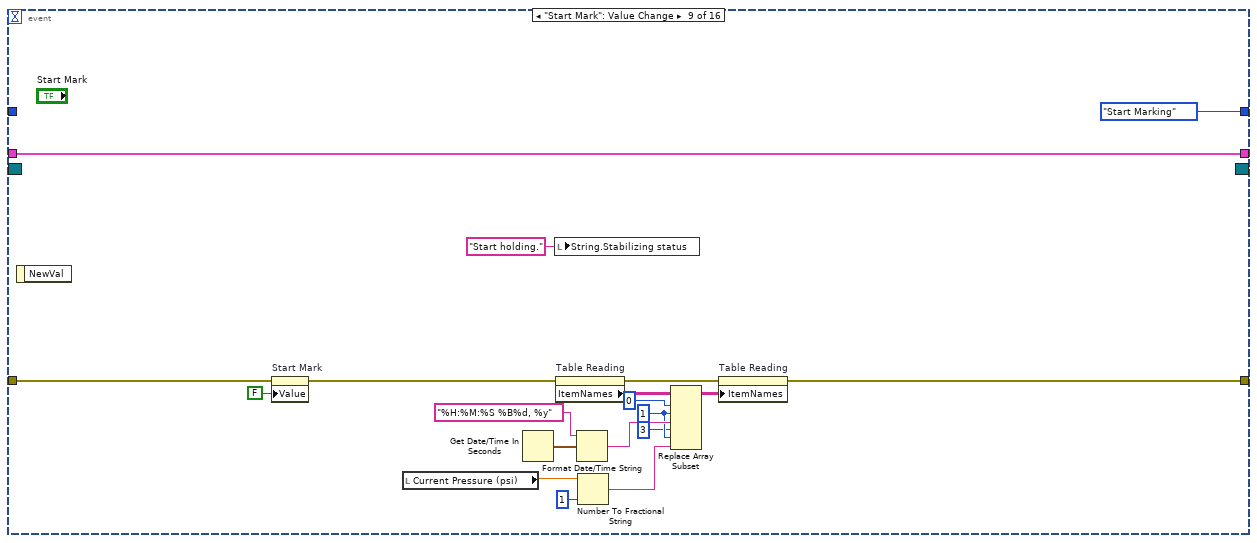
[diagram p20: hidden frame]
diagram:
  (unwired) Execute_-_Index_of_Elapse_time."Recording Duration"
  (unwired) Execute_-_Index_of_Elapse_time."Elapse Gap Data"
  w2 = Page_-_Execute_State."Init"
  # "Start Holding Pressure (psi)"
  # "End Holding Pressure (psi)"
  # "1.25"
  n1 = while {
    shift-right: [w7] -> _
    shift-left: w2 -> [w9]
    shift-right: [w10] -> _
    shift-left: errorcluster {"status"=FALSE, "code"=0, "source"=""} ("Error In") -> [w11]
    shift-right: [w5] -> _
    shift-left: T16 {"T_Out"=-1, "Point Phase"=[], "polar attributes"={"maximum"=0.0, "minimum"=0.0, "clip to min"=FALSE, "log?(F)"=FALSE, "grid color"=6710886, "plot color"=16711680, "fmt and prec"={"format"=enum."Decimal", "precision"=0}, "visible section"=8}, "Current Pressure"=0.0, "Counter Time"=0.0, "marking plot colour"=0, "Active Cursor"=0, "Event AI Data"=[], "Run Test"=FALSE, "Config"={"Holding Pressure"=0.0, "Set Polar Time"=0.0}, "Array of Elapse Time"=[], "Remaining Holding Time"=0.0, "Max Pressure"=0.0, "Start Mark"=FALSE, "Plot length (min)"=2.0, "Plot length scale"=3.0, "Magnitude ,y"=[], "Time ,x"=[], "Result Elapse"=[], "Phase"=[], "data array [mag, phase (deg)]"=[], "Max Phase"=0.0, "Plot and scale"={"Size Linear plot"=3, "Size point plot"=6, "Plot Scale"=0.2}, "Start Holding Pressure (psi)"=0.0, "End Holding Pressure (psi)"=0.0, "Marking Data"=[], "Display Polar Scale"={"Time Scale Label"="", "Max Scale label"=""}, "report out"=refnum, "axis labels"=["", "90", "180", "270"], "Polar Picture"=bytes[4090], "Event Ref"=refnum, "Data to Execute"={"Transaction Info"={"Transaction Number"="", "Order Number"="", "Quantity"=0, "Customer"=0, "Customer Description"="", "Project"="", "Sales Order"=0, "Material"="", "Material Description"="", "Rework"=FALSE, "NCR No."="", "Ref Order No."="", "Item No."=0, "BOM Rev."=0.0}, "Product Info"={"Product Category"="", "Procedure No./Ref."="", "Test System"="", "Test System Description"="", "Working Pressure"="", "Pressure Unit"="", "Rev."="", "PSL"=""}, "Misc - Additional Refs"=[], "Misc - Sensors"=[], "Misc - Tools"=[], "Acceptance Criteria Info"={"Max Start Hold Pressure"=0.0, "Enum.Max Start Hold Pressure"=enum."%", "Permitted Hold Pressure Drop"=0.0, "Enum.Permitted Hold Pressure Drop"=enum."%", "Pressure stabilize wait time"=10.0, "Enum.Pressure stabilize wait time"=enum."minutes"}, "Execution Info"={"Auto Set Marker"=FALSE, "Auto Stop Test"=FALSE}, "Results Info"={"ListBox.Output Set"="", "Output Set Description"=""}, "Notes"=""}, "Sequence Data"=[], "Holding Started?"=FALSE, "%Pressure Stabilized"=0.0, "Target Holding Time"=0.0, "Datalog path"=path "", "AI Offset"=[], "Sequence Number"=0, "Current Sequence"={"Seq.Select"=FALSE, "Seq.Status"=0, "Seq.Run"=FALSE, "Seq.TestSequence"=0.0, "Seq.No"=0.0, "Seq.ReqID"="", "Seq.TestReq"="", "Seq.Variance"="", "Seq.TestProcedure"="", "Seq.Section"="", "Seq.TestSystem"="", "Seq.TestPressure"="", "Seq.Cycle"="", "Seq.TestGroup"=0.0, "Seq.MSHP"=0.0, "Seq.PHPD"=0.0, "Seq.HoldingTime"="", "Seq.ChartScale"="", "Seq.ActuatorPressure"="", "Seq.MaxBDPressure"="", "Seq.BDIndicator"=FALSE, "Seq.TestMedia"=""}, "All Sequence Done"=TRUE, "Sequence Started"=FALSE, "Default View"="Polar Plot", "View Change Duration"=1.0, "First data point?"=TRUE, "Test Pressure Range"={"Maximum"=0.0, "Minimum"=0.0, "Pressure in range?"=FALSE}, "Stabilizing wait time"=0.0, "Run Pressure Data"={"Max Pressure"=0.0, "Min Pressure"=0.0, "Max Pressure TS"=timestamp(0 s since 1904-01-01), "Min Pressure TS"=timestamp(0 s since 1904-01-01)}, "Drop Rate Param"={"Drop Rate Calc Interval (sec)"=15.0, "Last Pressure (psi)"=0.0, "Allowable Press. Drop/min"=0.0, "Pressure Drop Accepted?"=FALSE, "Block interval to test"=10, "Block counter"=0, "Allowable Press. Drop/hr"=0.0}, "TestType"=enum."Holding", "Blowdown Param"={"Actuator Pressure"=0.0, "Max BD Pressure"=0.0, "BD Triggered"=FALSE, "BD Pressure"=0.0}} -> [w6]
    shift-left: w2 -> [w4]
    stop <- w8 stop-if-true
    # "This module"
    n2 = case shown="No Error" w11 {
      selector: w11 -> [w17 w1280]
      tunnel: w9 -> [w16 w1285]
      tunnel: [w18 w1281] -> w10
      tunnel: [w15 FALSE] -> w8
      tunnel: [w14 w1285] -> w7
      tunnel: w6 -> [w13 w1284]
      tunnel: [w12 w1284] -> w5
      tunnel: w4 -> [_ w1277]
      frame No Error {
        n3 = case shown="\"Calc. press. drop rate\"" w16 {
          selector: w16 -> [_ _ _ w118 _ _ _ _ _ _ _ _ _ _ _ _ _ _ _ _ _ _ _ _ _ _ _ _ _ _ _ _ _ _ _ _ _ _ _ _ _ _ _ _ _ _ _ w1274]
          tunnel: [w27 w65 w70 w123 w357 w418 w436 w485 w514 w534 w583 w610 w668 w708 w741 w760 w802 w819 w832 w834 w862 w876 w897 w920 w936 w965 w979 w1011 w1025 w1026 w1047 w1079 w1098 w1111 w1158 w1175 w1182 w1192 w1207 w1217 w1220 w1225 w1230 w1250 w1257 w1266 w1270 w1275] -> w18
          tunnel: w17 -> [w49 w53 w75 w122 w376 w428 w437 w485 w515 w535 w584 w610 w681 w708 w741 w760 w803 w819 w832 w835 w862 w876 w897 w921 w937 w968 w990 w1011 w1025 w1026 w1049 w1095 w1098 w1145 w1158 w1176 w1187 w1192 w1207 w1217 w1221 w1226 w1231 w1250 w1258 w1266 w1270 w1276]
          tunnel: [FALSE FALSE FALSE FALSE FALSE _ _ _ FALSE FALSE _ FALSE FALSE _ _ _ _ _ _ _ _ FALSE FALSE FALSE FALSE FALSE FALSE FALSE FALSE _ _ FALSE FALSE FALSE _ FALSE FALSE _ _ _ _ _ _ _ _ _ _ TRUE] -> w15
          tunnel: [Page_-_Execute_State."Register Event" Page_-_Execute_State."Idle" Page_-_Execute_State."Idle" w120 Page_-_Execute_State."Init File and Folder" Page_-_Execute_State."Idle" Page_-_Execute_State."Get pressure range" Page_-_Execute_State."Idle" Page_-_Execute_State."Idle" w530 w573 Page_-_Execute_State."Display Data" w674 w694 w730 Page_-_Execute_State."Calc. stabilizing elapsed time" Page_-_Execute_State."Calc. Max Min Pressure" Page_-_Execute_State."Polar attributes" Page_-_Execute_State."Idle" w838 Page_-_Execute_State."Polar attributes" Page_-_Execute_State."Insert Acc Data" Page_-_Execute_State."Convert Time To Phase" Page_-_Execute_State."Get Plot length" Page_-_Execute_State."Polar linear Plot" Page_-_Execute_State."Polar Point" Page_-_Execute_State."Display Label" Page_-_Execute_State."Plot linear Graph" w1013 Page_-_Execute_State."Display Holding Time" Page_-_Execute_State."Idle" Page_-_Execute_State."Finish Test" Page_-_Execute_State."Save  Data" Page_-_Execute_State."Get Next Sequence" w1156 Page_-_Execute_State."Fillup Report" Page_-_Execute_State."Idle" Page_-_Execute_State."Idle" Page_-_Execute_State."Update Info - Product" Page_-_Execute_State."Update Info - Additional Refs" Page_-_Execute_State."Update Info - Sensors" Page_-_Execute_State."Update Info - Tools" Page_-_Execute_State."Update Info - Acceptance Criteria" Page_-_Execute_State."Update Info - Execution" Page_-_Execute_State."Update Info - Results" Page_-_Execute_State."Update Info - Notes" Page_-_Execute_State."Get Current Sequence" w1274] -> w14
          tunnel: w13 -> [w47 w61 w67 w114 w379 w426 w461 w484 w512 w532 w579 w606 w665 w706 w735 w748 w791 w817 w831 w847 w859 w879 w910 w925 w951 w970 w977 w997 w1019 w1028 w1045 w1087 w1101 w1137 w1157 w1179 w1186 w1191 w1205 w1216 w1222 w1227 w1232 w1249 w1261 w1265 w1268 w1272]
          tunnel: [w43 w60 w66 w116 w378 w410 w434 w477 w511 w533 w577 w604 w665 w704 w734 w761 w791 w810 w831 w841 w860 w889 w903 w922 w947 w963 w975 w997 w1019 w1028 w1044 w1087 w1100 w1137 w1155 w1174 w1186 w1191 w1205 w1216 w1222 w1227 w1232 w1237 w1261 w1265 w1268 w1272] -> w12
          frame "Init", Default {
            w23 = FALSE ("Visible")
            w26 = "Polar Plot" ("Value (Signaling)")
            w39 = string[][] [["Start Holding Time & Date", ""], ["End Holding Time & Date", ""], ["Recorded Hold Time", ""], ["Start Holding Pressure (psi)", ""], ["End Holding Pressure (psi)", ""], ["Different in Holding Pressure, psi(%s)", ""], ["Permitted Holding Pressure Drop, psi(%)", ""], ["Test Status", ""], ["Recording duration (HH:MM:SS)", ""], ["Maximum pressure recorded (psi @ Time and Date)", ""], ["Minimum pressure recorded (psi @ Time and Date)", ""], ["Torque (Blowdown)", ""], ["Test performed by", ""], ["Test approved by", ""]] ("Item Names")
            w33 = 0.0 ("element")
            # "Init VI to default. Set HMI size"
            n4 = control-ref of="This VI"() -> (w45:refnum<vi>)
            n5 = call "Gen - Init to Default.vi"("Error in"=w49, "This VI"=w45) -> ("Error out"=w48:errorcluster, "This VI Copy"=w44:refnum<vi>)  [unwired: 8 in]
            n6 = call "Gen - Front Panel Size.vi"("Error In"=w48, "This VI"=w44) -> ("Error Out"=w41:errorcluster)  [unwired: 9 in]
            n7 = call "Get Enum Size.vi"("Enum"=Execute_-_Index_of_Elapse_time."Elapse Gap Data") -> ("Size"=w20:i32)
            n8 = Get Date/Time In Seconds() -> (seconds since 1Jan1904=w36:timestamp)
            n9 = Initialize Array(w36, w20) -> (w35:timestamp[])
            n10 = Initialize Array(w33, w20) -> (w32:dbl[])
            n11 = Initialize Array(w33, 4 ("dimension size")) -> (w34:dbl[])
            n12 = local write "Polar Plot"(picture bytes[9160] ("Polar Plot")) -> ()
            n13 = Bundle By Name(cluster=w47, "Array of Elapse Time"=w35, "Result Elapse"=w32, "AI Offset"=w34, "Drop Rate Param.Block interval to test"=4) -> (w43:T16)
            n14 = property on="Table Reading" class="MCListbox (strict)"(error in=w41, "ItemNames"=w39) -> (error out=w38:errorcluster)  [unwired: 1 in, 1 out]
            n15 = property on="Statistic" class="MCListbox (strict)"(error in=w38, "ItemNames"=w39) -> (error out=w37:errorcluster)  [unwired: 1 in, 1 out]
            n16 = property on="Indicator.PressureDropRatePsi" class="DigNum (strict)"("Visible"=w23) -> ()  [unwired: 2 in, 2 out]
            n17 = property on="Bool. Press Drop In Range" class="Bool (strict)"("Visible"=w23) -> ()  [unwired: 2 in, 2 out]
            n18 = local write "TabControl.TestType"(enum32{"Holding", "Blowdown"}."Holding" ("TabControl.TestType")) -> ()
            n19 = property on="View" class="CmbBox"(error in=w37, "Val(Sgnl)"=w26) -> (error out=w30:errorcluster)  [unwired: 1 in, 1 out]
            n20 = property on="View Change Duration" class="DigNum (strict)"(error in=w30, "Val(Sgnl)"=1.0 ("Value (Signaling)")) -> (error out=w28:errorcluster)  [unwired: 1 in, 1 out]
            n21 = property on="Default View" class="CmbBox"(error in=w28, "Val(Sgnl)"=w26) -> (error out=w27:errorcluster)  [unwired: 1 in, 1 out]
            "Test Status Ind" <- "Idle" ("Test Status Ind")
            "String.Stabilizing status" <- "" ("String.Stabilizing status")
          }
          frame "Register Event" {
            w52 = State_-_eFGV."Read" ("Action")
            # "Register all event"
            n22 = call "eFGV - Data to Execute.vi"("Action"=w52, "Error In"=w53) -> ("Error Out"=w54:errorcluster, "Event - Data to Execute"=w51:refnum<user-event>)  [unwired: 8 in]
            n23 = call "eFGV - Sequence Data.vi"("States"=w52, "Error In"=w54) -> ("Error Out"=w56:errorcluster, "Event - Sequence Data"=w55:refnum<user-event>)  [unwired: 7 in, 1 out]
            n24 = call "eFGV - AI Data.vi"("States"=w52, "Error In"=w56) -> ("Error Out"=w58:errorcluster, "Event AI Data"=w57:refnum<user-event>)  [unwired: 8 in]
            n25 = call "eFGV - Stop HMI.vi"("Action"=w52, "Error In"=w58) -> ("Error Out"=w64:errorcluster, "Event Stop HMI"=w62:refnum<user-event>)  [unwired: 7 in, 1 out]
            n26 = register-events(error in=w64, w62, w57, w55, w51) -> (reference out=w50:refnum<event-registration>, error out=w65:errorcluster)  [unwired: 1 in]
            n27 = Bundle By Name(cluster=w61, "Event Ref"=w50) -> (w60:T16)
          }
          frame "Read Config File" {
            n28 = call "aFGV - Read Write Config.vi"("State"=enum16{"Read", "Write", "Delete"}."Read", "Section"=Section."Config", "Error In"=w75) -> ("Error Out"=w71:errorcluster, "Data out"=w69:string[], "Key Names"=w68:string[])  [unwired: 6 in]
            n29 = for {
              shift-right: [w84] -> w70
              shift-left: w71 -> [w82]
              tunnel: w68 -> [w83] mode=indexing
              tunnel: w69 -> [w81] mode=indexing
              shift-right: [w78] -> w66
              shift-left: w67 -> [w79]
              n30 = call <vilib>:"Delimited String to 1D String Array.vi"("delimiter"=",", "delimited string"=w81) -> ("string array"=w80:string[])  [unwired: 9 in]
              n31 = case shown="\"Holding Pressure\"" w83 {
                tunnel: w82 -> [w86 w96 w99 w106 w112]
                tunnel: [w86 w96 w98 w106 w112] -> w84
                tunnel: w80 -> [_ w93 w97 w102 w109]
                tunnel: w79 -> [w85 w95 w100 w105 w111]
                tunnel: [w85 w95 w100 w104 w108] -> w78
                frame Default {
                }
                frame "Holding Pressure" {
                  n32 = Fract/Exp String To Number(string=w93) -> (number=w94:dbl[])  [unwired: 3 in, 1 out]
                  n33 = Index Array(array=w94) -> (element=w87:dbl)  [unwired: 1 in]
                  "Holding Pressure (psi)" <- w87
                  n34 = Multiply(x=w87, y=0.03) -> (x*y=w90:dbl)
                  n35 = Format Into String(format string="%.1f psi(%.1f %%)", w90, 3.0 ("input 2")) -> (resulting string=→"Permitted Holding Pressure Drop, psi%":string)  [unwired: 2 in, 1 out]
                }
                frame "Test Type" {
                  n36 = property on="Test Type" class="CmbBox"(error in=w99, "Strings[]"=w97) -> (error out=w98:errorcluster)  [unwired: 1 in, 1 out]
                }
                frame "Set Polar Time" {
                  n37 = Fract/Exp String To Number(string=w102) -> (number=w103:dbl[])  [unwired: 3 in, 1 out]
                  n38 = Index Array(array=w103) -> (element=w101:dbl)  [unwired: 1 in]
                  n39 = Bundle By Name(cluster=w105, "Config.Set Polar Time"=w101) -> (w104:T16)
                }
                frame "Holding Time" {
                  n40 = Fract/Exp String To Number(string=w109) -> (number=w110:dbl[])  [unwired: 3 in, 1 out]
                  n41 = Index Array(array=w110) -> (element=w107:dbl)  [unwired: 1 in]
                  n42 = Bundle By Name(cluster=w111, "Remaining Holding Time"=w107) -> (w108:T16)
                }
              }
            }
          }
          frame "Idle" {
            n43 = Unbundle By Name(w114) -> ("Event Ref"=w117:refnum<event-registration>)
            n44 = Unbundle By Name(w114) -> ("T_Out"=w113:i32)
            n45 = event shown="[11] \"End Mark\": Value Change" {
              selector: w117 -> [_ _ _ _ _ _ _ _ _ _ _ _ _ _ _ _]
              dyn-events: [_ _ _ _ _ _ _ _ _ _ _ _ _ _ _ _] -> w115
              timeout: w113 -> [_ _ _ _ _ _ _ _ _ _ _ _ _ _ _ _]
              tunnel: [w126 w136 w161 w178 w183 w187 w200 w211 w219 w239 w297 w305 w333 w350 w353 w356] -> w123
              tunnel: w122 -> [w126 w136 w161 w178 w183 w188 w200 w211 w234 w240 w297 w308 w339 w350 w353 w356]
              tunnel: [Page_-_Execute_State."Idle" w132 Page_-_Execute_State."Idle" Page_-_Execute_State."Update Info - Transaction" Page_-_Execute_State."Idle" Page_-_Execute_State."Idle" Page_-_Execute_State."Idle" w210 Page_-_Execute_State."Start Marking" w236 Page_-_Execute_State."Idle" Page_-_Execute_State."Idle" Page_-_Execute_State."Clear Mark" Page_-_Execute_State."Finish Test" w351 Page_-_Execute_State."Close"] -> w120
              tunnel: [w124 w129 w159 w176 w181 w190 w198 w202 w218 w238 w295 w328 w342 w349 w352 w355] -> w119
              tunnel: w114 -> [w124 w131 w162 w177 w182 w194 w199 w209 w218 w241 w296 w330 w344 w349 w352 w355]
              tunnel: w118 -> [_ _ _ _ _ _ _ _ _ _ _ _ _ _ w351 _]
              event Timeout {
                n46 = event-data() -> ()  [unwired: 1 in, 1 out]
              }
              event User Event {
                n47 = event-data() -> ("Event AI Data"=w135:sgl[])  [unwired: 1 in]
                n48 = Unbundle By Name(w131) -> ("First data point?"=w128:bool)
                n49 = Bundle By Name(cluster=w131, "Event AI Data"=w135) -> (w130:T16)
                n50 = case shown="False" w128 {
                  tunnel: w130 -> [w143 w148]
                  tunnel: [w141 w153] -> w129
                  frame True {
                    n51 = Unbundle By Name(w143) -> ("Array of Elapse Time"=w142:timestamp[])
                    n52 = Get Date/Time In Seconds() -> (seconds since 1Jan1904=w138:timestamp)
                    n53 = Replace Array Subset(array=w142, new element=w138, index=Execute_-_Index_of_Elapse_time."Elapse Gap Data") -> (w140:timestamp[])
                    n54 = Bundle By Name(cluster=w143, "Array of Elapse Time"=w140, "First data point?"=FALSE) -> (w141:T16)
                  }
                  frame False {
                    w145 = Execute_-_Index_of_Elapse_time."Elapse Gap Data"
                    n55 = Unbundle By Name(w148) -> ("Array of Elapse Time"=w151:timestamp[])
                    n56 = Unbundle By Name(w148) -> ("Result Elapse"=w147:dbl[])
                    n57 = Index Array(array=w151, index=w145) -> (element=w149:timestamp)
                    n58 = Get Date/Time In Seconds() -> (seconds since 1Jan1904=w150:timestamp)
                    n59 = Subtract(x=w150, y=w149) -> (x-y=w144:dbl)
                    n60 = Replace Array Subset(array=w151, new element=w150, index=w145) -> (w152:timestamp[])
                    n61 = Replace Array Subset(array=w147, new element=w144, index=w145) -> (w146:dbl[])
                    n62 = Bundle By Name(cluster=w148, "Array of Elapse Time"=w152, "Result Elapse"=w146) -> (w153:T16)
                  }
                }
                n63 = Unbundle By Name(w129) -> ("Sequence Started"=w134:bool)
                n64 = Select(t=Page_-_Execute_State."Get Current Pressure", s=w134, f=Page_-_Execute_State."Idle") -> (s? t:f=w132:T17)
              }
              event User Event {
                n65 = event-data() -> ("Sequence Data"=w158:T13[])  [unwired: 1 in]
                n66 = call "Sort Sequence List.vi"("Sequence Data In"=w158) -> ("Sequence Data Out"=w157:T13[])
                n67 = for {
                  tunnel: w157 -> [w165] mode=indexing
                  tunnel: [w163] -> w156 mode=indexing
                  n68 = Bundle By Name(cluster=w165, "Seq.Status"=u32 16711680) -> (w163:T13)
                }
                n69 = local write "Sequence List"(w156) -> ()
                n70 = Bundle By Name(cluster=w162, "Sequence Data"=w156, "All Sequence Done"=FALSE, "Sequence Number"=0) -> (w159:T16)
              }
              event User Event {
                n71 = event-data() -> ("Transaction Info"=w175:T8, "Product Info"=w174:T9, "Misc - Additional Refs"=w173:string[][], "Misc - Sensors"=w172:string[][], "Misc - Tools"=w171:string[][], "Acceptance Criteria Info"=w170:T10, "Execution Info"=w169:T11, "Results Info"=w168:T12, "Notes"=w167:string)  [unwired: 1 in]
                n72 = Bundle By Name(cluster=w177, "Data to Execute.Transaction Info"=w175, "Data to Execute.Product Info"=w174, "Data to Execute.Misc - Additional Refs"=w173, "Data to Execute.Misc - Sensors"=w172, "Data to Execute.Misc - Tools"=w171, "Data to Execute.Acceptance Criteria Info"=w170, "Data to Execute.Execution Info"=w169, "Data to Execute.Results Info"=w168, "Data to Execute.Notes"=w167) -> (w176:T16)
              }
              event "Default View": Value Change {
                n73 = event-data() -> ("NewVal"=w180:string)  [unwired: 1 in]
                n74 = Bundle By Name(cluster=w182, "Default View"=w180) -> (w181:T16)
              }
              event "View": Value Change {
                n75 = event-data() -> ("NewVal"=w186:string)  [unwired: 1 in]
                n76 = Unbundle By Name(w194) -> ("Array of Elapse Time"=w193:timestamp[])
                n77 = Get Date/Time In Seconds() -> (seconds since 1Jan1904=w192:timestamp)
                n78 = Replace Array Subset(array=w193, new element=w192, index=Execute_-_Index_of_Elapse_time."View Change") -> (w189:timestamp[])
                n79 = Bundle By Name(cluster=w194, "Array of Elapse Time"=w189) -> (w190:T16)
                n80 = Scan From String(input string=w186, default 1=T1."Key Value" ("tab - View Data")) -> (output 1=w184:T1)  [unwired: 3 in, 3 out]
                n81 = property on="tab - View Data" class="TabCtl (strict)"(error in=w188, "Value"=w184) -> (error out=w187:errorcluster)  [unwired: 1 in, 1 out]
              }
              event "View Change Duration": Value Change {
                n82 = event-data() -> ("NewVal"=w197:dbl)  [unwired: 1 in]
                n83 = Bundle By Name(cluster=w199, "View Change Duration"=w197) -> (w198:T16)
              }
              event "Start Test": Value Change {
                n84 = event-data() -> ("NewVal"=w201:bool)  [unwired: 1 in]
                n85 = Unbundle By Name(w209) -> ("All Sequence Done"=w207:bool, "Sequence Started"=w203:bool)
                n86 = Select(t=Page_-_Execute_State."Display Result Test" ("f"), s=w203, f=Page_-_Execute_State."Idle") -> (s? t:f=w204:T17)
                n87 = Bundle By Name(cluster=w209, "Run Test"=w201) -> (w202:T16)
                n88 = case shown="False" w207 {
                  tunnel: [Page_-_Execute_State."Init Test Param" Page_-_Execute_State."Idle"] -> w208
                  frame False {
                  }
                  frame True {
                    n89 = property on="Start Test" class="Bool (strict)"("Value"=FALSE ("Run Test")) -> ()  [unwired: 2 in, 2 out]
                    n90 = call "Gen - Popup Single Button (Auto Close).vi"("Message in"="All test sequence are done", "Header"="TEST SEQUENCE") -> ()  [unwired: 8 in, 2 out]
                  }
                }
                n91 = Select(t=w208, s=w201, f=w204) -> (s? t:f=w210:T17)
              }
              event "Start Mark": Value Change {
                w223 = 1 ("disabled index (col)")
                n92 = event-data() -> ()  [unwired: 1 in, 1 out]
                n93 = property on="Start Mark" class="Bool (strict)"(error in=w234, "Value"=FALSE ("Start Mark")) -> (error out=w220:errorcluster)  [unwired: 1 in, 1 out]
                n94 = local read "Current Pressure (psi)"() -> (w227:sgl)
                n95 = Get Date/Time In Seconds() -> (seconds since 1Jan1904=w232:timestamp)
                n96 = local write "String.Stabilizing status"("Start holding." ("String.Stabilizing status")) -> ()
                n97 = property on="Table Reading" class="MCListbox (strict)"(error in=w220) -> (error out=w228:errorcluster, "ItemNames"=w231:string[][])  [unwired: 1 in, 1 out]
                n98 = Format Date/Time String(time format string (%c)="%H:%M:%S %B%d, %y", seconds (now)=w232) -> (date/time string=w229:string)  [unwired: 1 in]
                n99 = Number To Fractional String(number=w227, precision (6)=i16 1) -> (F-format string=w226:string)  [unwired: 2 in]
                n100 = Replace Array Subset(array=w231, new element #1=w229, index (row) #1=0 ("disabled index (row)"), index (col) #1=w223, new element #2=w226, index (row) #2=3 ("index (row)"), index (col) #2=w223) -> (w230:string[][])
                n101 = property on="Table Reading" class="MCListbox (strict)"(error in=w228, "ItemNames"=w230) -> (error out=w219:errorcluster)  [unwired: 1 in, 1 out]
              }
              event "Holding Started": Value Change {
                n102 = event-data() -> ("NewVal"=w237:bool)  [unwired: 1 in, 5 out]
                n103 = case shown="True" w237 {
                  selector: w237 -> [w249 w274]
                  tunnel: w241 -> [w250 w275]
                  tunnel: w240 -> [w243 w276]
                  tunnel: [w242 w291] -> w239
                  tunnel: [w245 w290] -> w238
                  tunnel: [w244 Page_-_Execute_State."Idle"] -> w236
                  frame False {
                    n104 = local read "Hold Time Remainder"() -> (w247:dbl)
                    n105 = Bundle By Name(cluster=w250, "Holding Started?"=w249) -> (w246:T16)
                    n106 = Greater Than 0?(x=w247) -> (x > 0?=w248:bool)
                    n107 = case shown="True" w248 {
                      tunnel: w246 -> [w253 w265]
                      tunnel: [w253 w263] -> w245
                      tunnel: [Page_-_Execute_State."Idle" Page_-_Execute_State."Get Next Sequence"] -> w244
                      tunnel: w243 -> [w251 w256]
                      tunnel: [w251 w254] -> w242
                      frame False {
                      }
                      frame True {
                        w257 = "Failed" ("Test Status Ind")
                        n108 = Unbundle By Name(w265) -> ("Sequence Data"=w268:T13[], "Sequence Number"=w266:i32)
                        n109 = property on="Table Reading" class="MCListbox (strict)"(error in=w256) -> (error out=w255:errorcluster, "ItemNames"=w261:string[][])  [unwired: 1 in, 1 out]
                        n110 = local write "Test Status Ind"(w257) -> ()
                        n111 = Index Array(array=w268, index=w266) -> (element=w270:T13)
                        n112 = Replace Array Subset(array=w261, new element=w257, index (row)=7, index (col)=1 ("disabled index (col)")) -> (w260:string[][])
                        n113 = Bundle By Name(cluster=w270, "Seq.Status"=u32 13816530) -> (w267:T13)
                        n114 = property on="Table Reading" class="MCListbox (strict)"(error in=w255, "ItemNames"=w260) -> (error out=w254:errorcluster)  [unwired: 1 in, 1 out]
                        n115 = Replace Array Subset(array=w268, new element=w267, index=w266) -> (w262:T13[])
                        n116 = Bundle By Name(cluster=w265, "Sequence Data"=w262) -> (w263:T16)
                        n117 = local write "Sequence List"(w262) -> ()
                        n118 = call "Gen - Popup Single Button (Auto Close).vi"("Type"=enum16{"Error", "Info"}."Error", "Message in"="Pressure Drops Below Allowable Range before test finishes.\nMoving to next sequence", "Header"="HOLDING TIME") -> ()  [unwired: 7 in, 2 out]
                      }
                    }
                  }
                  frame True {
                    n119 = local read "Hold Time (hh:mm)"() -> (w289:string)
                    n120 = call <vilib>:"Delimited String to 1D String Array.vi"("delimiter"=":", "delimited string"=w289) -> ("string array"=w287:string[])  [unwired: 9 in]
                    n121 = Index Array(array=w287) -> (element #1=w286:string, element #2=w285:string)  [unwired: 2 in]
                    n122 = Decimal String To Number(string=w286) -> (number=w284:i32)  [unwired: 2 in, 1 out]
                    n123 = Decimal String To Number(string=w285) -> (number=w281:i32)  [unwired: 2 in, 1 out]
                    n124 = Multiply(x=3600, y=w284) -> (x*y=w282:i32)
                    n125 = Multiply(x=60, y=w281) -> (x*y=w279:i32)
                    n126 = Add(x=w282, y=w279) -> (x+y=w278:i32)
                    n127 = Bundle By Name(cluster=w275, "Remaining Holding Time"=w278, "Target Holding Time"=w278, "Holding Started?"=w274) -> (w290:T16)
                    n128 = property on="Start Mark" class="Bool (strict)"(error in=w276, "Val(Sgnl)"=w274) -> (error out=w291:errorcluster)  [unwired: 1 in, 1 out]
                  }
                }
              }
              event "TARE": Value Change {
                n129 = event-data() -> ()  [unwired: 1 in, 1 out]
                n130 = Unbundle By Name(w296) -> ("Event AI Data"=w293:sgl[])
                n131 = Negate(x=w293) -> (-x=w292:sgl[])
                n132 = Bundle By Name(cluster=w296, "AI Offset"=w292) -> (w295:T16)
              }
              event "End Mark": Value Change {
                w311 = 1 ("disabled index (col)")
                w323 = u32 1 ("Active Cursor")
                n133 = event-data() -> ()  [unwired: 1 in, 1 out]
                n134 = local read "Current Pressure (psi)"() -> (w314:sgl)
                n135 = Unbundle By Name(w330) -> ("Counter Time"=w321:dbl, "Point Phase"=w329:dbl[], "Current Pressure"=w320:sgl)
                n136 = Get Date/Time In Seconds() -> (seconds since 1Jan1904=w319:timestamp)
                n137 = property on="Table Reading" class="MCListbox (strict)"(error in=w308) -> (error out=w315:errorcluster, "ItemNames"=w318:string[][])  [unwired: 1 in, 1 out]
                n138 = Format Date/Time String(time format string (%c)="%H:%M:%S %B%d, %Y", seconds (now)=w319) -> (date/time string=w316:string)  [unwired: 1 in]
                n139 = Number To Fractional String(number=w314, precision (6)=i16 1) -> (F-format string=w313:string)  [unwired: 2 in]
                n140 = Replace Array Subset(array=w318, new element #1=w316, index (row) #1=1 ("disabled index (row)"), index (col) #1=w311, new element #2=w313, index (row) #2=4 ("index (row)"), index (col) #2=w311) -> (w317:string[][])
                n141 = property on="Table Reading" class="MCListbox (strict)"(error in=w315, "ItemNames"=w317) -> (error out=w307:errorcluster)  [unwired: 1 in, 1 out]
                n142 = local write "String.Stabilizing status"("Holding ended." ("String.Stabilizing status")) -> ()
                n143 = Insert Into Array(array=w329, new element=w321) -> (w327:dbl[])  [unwired: 1 in]
                n144 = Bundle By Name(cluster=T19 {"X"=0.0, "Y"=0.0} ("Cursor.Cursor Position"), "Y"=w320, "X"=w321) -> (w325:T19)
                n145 = property on="Linear Graph" class="XYGraph (strict)"(error in=w307, "Active Cursor"=w323, "Cursor.Cursor Color"="Stop Marker", "Cursor.Cursor Position"=w325, "Cursor.Visible"=TRUE) -> (error out=w299:errorcluster)  [unwired: 1 in, 1 out]
                n146 = local read "Blow Down  Test"() -> (w301:bool)
                n147 = Select(t=Control_1."Blowdown" ("TestType"), s=w301, f=Control_1."Holding") -> (s? t:f=w300:T15)
                n148 = Bundle By Name(cluster=w330, "Point Phase"=w327, "marking plot colour"="Stop Marker", "Active Cursor"=w323, "TestType"=w300) -> (w328:T16)
                n149 = local write "TabControl.TestType"(w300) -> ()
                n150 = property on="End Mark" class="Bool (strict)"(error in=w299, "Value"=FALSE ("End Mark")) -> (error out=w305:errorcluster)  [unwired: 1 in, 1 out]
              }
              event "Clear Mark": Value Change {
                n151 = event-data() -> ()  [unwired: 1 in, 1 out]
                n152 = Unbundle By Name(w344) -> ("Point Phase"=w343:dbl[], "Active Cursor"=w337:u32)
                n153 = Reverse 1D Array(array=w343) -> (reversed array=w347:dbl[])
                n154 = Delete From Array(array=w347, length=1, index=0) -> (array with subset deleted=w335:dbl[])  [unwired: 1 out]
                n155 = property on="Linear Graph" class="XYGraph (strict)"(error in=w339, "Active Cursor"=w337, "Cursor.Visible"=FALSE) -> (error out=w334:errorcluster)  [unwired: 1 in, 1 out]
                n156 = Reverse 1D Array(array=w335) -> (reversed array=w341:dbl[])
                n157 = Bundle By Name(cluster=w344, "Point Phase"=w341, "Start Mark"=FALSE) -> (w342:T16)
                n158 = property on="Clear Mark" class="Bool"(error in=w334, "Value"=FALSE) -> (error out=w333:errorcluster)  [unwired: 1 in, 1 out]
              }
              event "Finish": Value Change {
                n159 = event-data() -> ()  [unwired: 1 in, 6 out]
              }
              event "Stop": Value Change {
                n160 = event-data() -> ()  [unwired: 1 in, 6 out]
              }
              event User Event {
                n161 = event-data() -> ()  [unwired: 1 in, 5 out]
              }
            }
            n162 = Bundle By Name(cluster=w119, "Event Ref"=w115) -> (w116:T16)
          }
          frame "Init Test Param" {
            w373 = sgl[] [] ("Magnitude ,y")
            n163 = Unbundle By Name(w379) -> ("Array of Elapse Time"=w383:timestamp[], "Config.Holding Pressure"=w371:dbl)
            n164 = property on="Recording Duration" class="Str"(error in=w376, "Value"="00:00:00" ("Recording Duration")) -> (error out=w375:errorcluster)  [unwired: 1 in, 1 out]
            n165 = Get Date/Time In Seconds() -> (seconds since 1Jan1904=w359:timestamp)
            n166 = Multiply(x=w371, y=1.25) -> (x*y=w369:dbl)
            n167 = for {
              N: 2 -> [_]
              tunnel: [w392] -> w358
              tunnel: w375 -> [w389]
              tunnel: w369 -> [w388]
              i -> [w391]
              n168 = property on="Linear Graph" class="XYGraph (strict)"(error in=w389, "Active Cursor"=w391, "Cursor.Visible"=FALSE, "YScale.Maximum"=w388) -> (error out=w392:errorcluster)  [unwired: 1 in, 1 out]
            }
            n169 = Replace Array Subset(array=w383, new element #1=w359, index #1=Execute_-_Index_of_Elapse_time."Elapse Gap Data", new element #2=w359, index #2=Execute_-_Index_of_Elapse_time."Recording Duration", new element #3=w359, index #3=Execute_-_Index_of_Elapse_time."Press. Drop Rate") -> (w384:timestamp[])
            n170 = local write "String.Stabilizing status"("Pressure not in range" ("String.Stabilizing status")) -> ()
            n171 = disable-structure shown="Enabled" {
              disable-tunnel: w358 -> [w387 _]
              disable-tunnel: [w386 _] -> w357
              frame Enabled {
                n172 = property on="TARE" class="Bool (strict)"(error in=w387, "Val(Sgnl)"=FALSE ("Value (Signaling)")) -> (error out=w386:errorcluster)  [unwired: 1 in, 1 out]
              }
              frame Disabled {
              }
            }
            n173 = Get Date/Time In Seconds() -> (seconds since 1Jan1904=w364:timestamp)
            n174 = Bundle By Name(cluster=w379, "Array of Elapse Time"=w384, "Counter Time"=0.0 ("Counter"), "Magnitude ,y"=w373, "Time ,x"=w373, "Run Test"=TRUE, "Start Mark"=FALSE, "T_Out"=-1, "Point Phase"=dbl[] [], "First data point?"=TRUE, "Run Pressure Data.Min Pressure TS"=w364) -> (w378:T16)
          }
          frame "Init File and Folder" {
            w394 = "Testing" ("Test Status Ind")
            n175 = Unbundle By Name(w426) -> ("Current Sequence.Seq.No"=w406:dbl, "Data to Execute.Transaction Info.Transaction Number"=w393:string)
            n176 = call "FGV - Data Path.vi"("FGV State"=State_-_FGV."Read", "Error In"=w428) -> ("Error Out"=w404:errorcluster, "Path Out"=w425:path)  [unwired: 8 in]
            n177 = Build Path(base path=w425, name or relative path=path "Results") -> (appended path=w423:path)
            n178 = Build Path(base path=w423, name or relative path=w393) -> (appended path=w408:path)
            n179 = Concatenate Strings("SeqNo" ("string"), w406) -> (w405:string)
            "SequenceNoFolder" <- w405
            n180 = Build Path(base path=w408, name or relative path=w405) -> (appended path=w402:path)
            n181 = Create Folder(path (use dialog)=w402, error in=w404) -> (created path=w401:path, error out=w403:errorcluster)  [unwired: 1 in, 1 out]
            n182 = Build Path(base path=w401, name or relative path=path "Data.csv") -> (appended path=w417:path)
            n183 = Unbundle By Name(w426) -> ("Sequence Data"=w413:T13[], "Sequence Number"=w411:i32)
            n184 = Index Array(array=w413, index=w411) -> (element=w415:T13)
            n185 = Bundle By Name(cluster=w415, "Seq.Status"=u32 3381759) -> (w412:T13)
            n186 = property on="Table Reading" class="MCListbox (strict)"() -> ("ItemNames"=w398:string[][])  [unwired: 2 in, 2 out]
            n187 = local write "Test Status Ind"(w394) -> ()
            n188 = Replace Array Subset(array=w413, new element=w412, index=w411) -> (w399:T13[])
            n189 = call-poly <vilib>:"Write Delimited Spreadsheet.vi"("file path (dialog if empty)"=w417, "1D data"=string[] ["Timestamp", "Pressure 1", "Pressure 2", "Pressure 3", "Pressure 4"], "append to file? (new file:F)"=FALSE, "error in (no error)"=w403, "delimiter (\\t)"="," ("delimiter (\\t)")) -> ("new file path (Not A Path if cancelled)"=w409:path, "error out"=w418:errorcluster)  [unwired: 9 in]
            n190 = Replace Array Subset(array=w398, new element=w394, index (row)=7, index (col)=1 ("disabled index (col)")) -> (w397:string[][])
            n191 = local write "Sequence List"(w399) -> ()
            n192 = property on="Table Reading" class="MCListbox (strict)"("ItemNames"=w397) -> ()  [unwired: 2 in, 2 out]
            n193 = Bundle By Name(cluster=w426, "Sequence Data"=w399, "Datalog path"=w409, "Sequence Started"=TRUE) -> (w410:T16)
          }
          frame "Get Current Sequence" {
            w450 = FALSE ("Run Test")
            n194 = Unbundle By Name(w461) -> ("Sequence Data"=w460:T13[], "Sequence Number"=w459:i32)
            n195 = Index Array(array=w460, index=w459) -> (element=w433:T13)
            n196 = Bundle By Name(cluster=w461, "Current Sequence"=w433, "Run Test"=w450, "Sequence Started"=w450) -> (w449:T16)
            n197 = Unbundle By Name(w433) -> ("Seq.TestSequence"=→"Test Sequence":dbl, "Seq.No"=→"Seq.No":dbl, "Seq.TestReq"=→"Test Requirement":string, "Seq.Variance"=→"Variance":string, "Seq.TestMedia"=→"Test Media":string, "Seq.TestPressure"=w464:string, "Seq.HoldingTime"=→"Hold Time (hh:mm)":string, "Seq.BDIndicator"=w463:bool)  [unwired: 4 out]
            n198 = Decimal String To Number(string=w464) -> (number=w446:i32)  [unwired: 2 in, 1 out]
            "Test Pressure" <- w446
            n199 = Equal?(x=w463, y="Y") -> (x = y?=→"Blow Down  Test":bool)
            n200 = Unbundle By Name(w433) -> ("Seq.ActuatorPressure"=w432:string, "Seq.MaxBDPressure"=w431:string)
            n201 = Unbundle By Name(w449) -> ("Data to Execute.Acceptance Criteria Info.Permitted Hold Pressure Drop"=w441:dbl)
            n202 = Fract/Exp String To Number(string=w432) -> (number=w429:dbl)  [unwired: 3 in, 1 out]
            n203 = Fract/Exp String To Number(string=w431) -> (number=w430:dbl)  [unwired: 3 in, 1 out]
            n204 = Bundle By Name(cluster=w449, "Blowdown Param.Actuator Pressure"=w429, "Blowdown Param.Max BD Pressure"=w430) -> (w434:T16)
            n205 = Divide(x=w441, y=100.0) -> (x/y=w447:dbl)
            n206 = Multiply(x=w447, y=w446) -> (x*y=w442:dbl)
            n207 = Format Into String(format string="%.1f(%d%%)", w442, w441) -> (resulting string=w438:string)  [unwired: 2 in, 1 out]
            n208 = property on="Table Reading" class="MCListbox (strict)"(error in=w437) -> (error out=w435:errorcluster, "ItemNames"=w445:string[][])  [unwired: 1 in, 1 out]
            n209 = Replace Array Subset(array=w445, new element=w438, index (row)=6, index (col)=1 ("disabled index (col)")) -> (w444:string[][])
            n210 = property on="Table Reading" class="MCListbox (strict)"(error in=w435, "ItemNames"=w444) -> (error out=w436:errorcluster)  [unwired: 1 in, 1 out]
          }
          frame "Get pressure range" {
            n211 = Unbundle By Name(w484) -> ("Current Sequence.Seq.TestPressure"=w483:string, "Data to Execute.Acceptance Criteria Info.Max Start Hold Pressure"=w479:dbl, "Data to Execute.Acceptance Criteria Info.Enum.Max Start Hold Pressure"=w482:enum16{"%", "psi"}, "Test Pressure Range"=w481:T28, "Data to Execute.Acceptance Criteria Info.Pressure stabilize wait time"=w473:dbl, "Data to Execute.Acceptance Criteria Info.Enum.Pressure stabilize wait time"=w475:enum16{"seconds", "minutes"}, "Data to Execute.Acceptance Criteria Info.Enum.Permitted Hold Pressure Drop"=w471:enum16{"%", "psi"}, "Data to Execute.Acceptance Criteria Info.Permitted Hold Pressure Drop"=w470:dbl, "Current Sequence.Seq.TestPressure"=w469:string)
            n212 = Decimal String To Number(string=w483) -> (number=w480:i32)  [unwired: 2 in, 1 out]
            n213 = case shown="\"psi\"" w471 {
              tunnel: w470 -> [w490 w492]
              tunnel: [w486 w492] -> w465
              tunnel: w469 -> [w491 _]
              frame "%", Default {
                n214 = Fract/Exp String To Number(string=w491) -> (number=w487:dbl)  [unwired: 3 in, 1 out]
                n215 = Divide(x=w490, y=100.0) -> (x/y=w488:dbl)
                n216 = Multiply(x=w488, y=w487) -> (x*y=w486:dbl)
              }
              frame "psi" {
              }
            }
            n217 = case shown="\"seconds\", Default" w475 {
              tunnel: [1.0 60.0] -> w474
              frame "seconds", Default {
              }
              frame "minutes" {
              }
            }
            n218 = case shown="\"%\", Default" w482 {
              tunnel: w481 -> [w499 w510]
              tunnel: w480 -> [w497 w507]
              tunnel: w479 -> [w504 w509]
              tunnel: [w496 w506] -> w476
              frame "%", Default {
                n219 = Divide(x=w504, y=100.0) -> (x/y=w502:dbl)
                n220 = Add(x=1.0, y=w502) -> (x+y=w500:dbl)
                n221 = Multiply(x=w497, y=w500) -> (x*y=w498:dbl)
                n222 = Bundle By Name(cluster=w499, "Minimum"=w497, "Maximum"=w498, "Pressure in range?"=FALSE) -> (w496:T28)
              }
              frame "psi" {
                n223 = Add(x=w507, y=w509) -> (x+y=w508:dbl)
                n224 = Bundle By Name(cluster=w510, "Minimum"=w507, "Maximum"=w508, "Pressure in range?"=FALSE) -> (w506:T28)
              }
            }
            n225 = Multiply(x=w473, y=w474) -> (x*y=w472:dbl)
            n226 = Divide(x=w465, y=60.0) -> (x/y=w467:dbl)
            n227 = local read "Current Pressure (psi)"() -> (w466:sgl)
            n228 = Bundle By Name(cluster=w484, "Test Pressure Range"=w476, "Stabilizing wait time"=w472, "Drop Rate Param.Allowable Press. Drop/min"=w467, "Drop Rate Param.Last Pressure (psi)"=w466, "Drop Rate Param.Allowable Press. Drop/hr"=w465) -> (w477:T16)
          }
          frame "Clear Mark" {
            n229 = Unbundle By Name(w512) -> ("Point Phase"=w518:dbl[])
            n230 = Array Size(array=w518) -> (size(s)=w517:i32)
            n231 = Not Equal?(x=w517, y=1) -> (x != y?=w513:bool)
            n232 = case shown="False" w513 {
              tunnel: w515 -> [w521 w529]
              tunnel: [w521 w529] -> w514
              tunnel: w512 -> [w525 w528]
              tunnel: [w527 w528] -> w511
              frame False {
                n233 = Unbundle By Name(w525) -> ("Array of Elapse Time"=w524:timestamp[])
                n234 = Get Date/Time In Seconds() -> (seconds since 1Jan1904=w522:timestamp)
                n235 = Replace Array Subset(array=w524, new element=w522, index=Execute_-_Index_of_Elapse_time."Holding Time") -> (w526:timestamp[])
                n236 = Bundle By Name(cluster=w525, "Array of Elapse Time"=w526) -> (w527:T16)
              }
              frame True {
              }
            }
          }
          frame "Start Marking" {
            n237 = Unbundle By Name(w532) -> ("Start Mark"=w531:bool)
            n238 = case shown="True" w531 {
              tunnel: [w538 w565] -> w533
              tunnel: [w537 w544] -> w534
              tunnel: [Page_-_Execute_State."Idle" Page_-_Execute_State."Idle"] -> w530
              tunnel: w535 -> [w537 w552]
              tunnel: w532 -> [w538 w551]
              frame True {
              }
              frame False {
                w561 = u32 0 ("Active Cursor")
                n239 = Unbundle By Name(w551) -> ("Array of Elapse Time"=w550:timestamp[], "Point Phase"=w547:dbl[], "Counter Time"=w543:dbl, "Current Pressure"=w540:sgl)
                n240 = Insert Into Array(array=w547, new element=w543) -> (w564:dbl[])  [unwired: 1 in]
                n241 = Bundle By Name(cluster=T19 {"X"=0.0, "Y"=0.0} ("Cursor.Cursor Position"), "Y"=w540, "X"=w543) -> (w563:T19)
                n242 = Get Date/Time In Seconds() -> (seconds since 1Jan1904=w558:timestamp)
                n243 = property on="Linear Graph" class="XYGraph (strict)"(error in=w552, "Active Cursor"=w561, "Cursor.Cursor Color"="Start Marker", "Cursor.Cursor Position"=w563, "Cursor.Visible"=TRUE) -> (error out=w545:errorcluster)  [unwired: 1 in, 1 out]
                n244 = To Long Integer(number=Execute_-_Index_of_Elapse_time."Holding Time") -> (32bit integer=w549:i32)
                n245 = Replace Array Subset(array=w550, new element=w558, index=w549) -> (w557:timestamp[])
                n246 = Get Date/Time In Seconds() -> (seconds since 1Jan1904=w554:timestamp)
                n247 = Format Date/Time String(time format string (%c)="%d.%B.%Y %H:%M:%S" ("format string"), seconds (now)=w554) -> (date/time string=→"Start Holding Datetime":string)  [unwired: 1 in]
                n248 = Format Into String(format string="%.1f", error in=w545, w540) -> (resulting string=→"Start Holding Pressure (psi)":string, error out=w544:errorcluster)  [unwired: 1 in]
                n249 = Bundle By Name(cluster=w551, "Start Mark"=TRUE, "Array of Elapse Time"=w557, "Point Phase"=w564, "marking plot colour"="Start Marker", "Active Cursor"=w561, "Start Holding Pressure (psi)"=w540) -> (w565:T16)
              }
            }
          }
          frame "Get Current Pressure" {
            n250 = Unbundle By Name(w579) -> ("Event AI Data"=w592:sgl[], "AI Offset"=w591:sgl[])
            n251 = Add(x=w592, y=w591) -> (x+y=w589:sgl[])
            n252 = Index Array(array=w589, index #1=0 ("index"), index #2=1 ("index")) -> (element #1=w578:sgl, element #2=→"NumInd.2nd_pump_press":sgl)
            "Current Pressure (psi)" <- w578
            "Key Value Current Pressure (psi)" <- w578
            n253 = for {
              tunnel: w589 -> [w603] mode=indexing
              tunnel: [w602] -> w585 mode=indexing
              n254 = Number To Fractional String(number=w603, precision (6)=i16 1) -> (F-format string=w602:string)  [unwired: 2 in]
            }
            n255 = Bundle By Name(cluster=w579, "Current Pressure"=w578) -> (w577:T16)
            n256 = Get Date/Time In Seconds() -> (seconds since 1Jan1904=w588:timestamp)
            n257 = Format Date/Time String(time format string (%c)="%d/%m/%Y %H:%M:%S", seconds (now)=w588) -> (date/time string=w586:string)  [unwired: 1 in]
            n258 = Unbundle By Name(w577) -> ("Datalog path"=w582:path, "Run Test"=w580:bool)
            n259 = Unbundle By Name(w577) -> ("TestType"=w576:T15)
            n260 = Build Array (concatenate)(w586, w585) -> (w581:string[])
            n261 = case shown="True" w580 {
              tunnel: w584 -> [w593 w597]
              tunnel: [w593 w596] -> w583
              tunnel: w582 -> [_ w595]
              tunnel: w581 -> [_ w594]
              frame False {
              }
              frame True {
                n262 = call-poly <vilib>:"Write Delimited Spreadsheet.vi"("file path (dialog if empty)"=w595, "format (%s)"="%s" ("format (%.3f)"), "1D data"=w594, "append to file? (new file:F)"=TRUE, "error in (no error)"=w597, "delimiter (\\t)"="," ("delimiter (\\t)")) -> ("error out"=w596:errorcluster)  [unwired: 8 in, 1 out]
              }
            }
            n263 = Equal?(x=Control_1."Holding", y=w576) -> (x = y?=w568:bool)
            n264 = Select(t="Holding Test" ("Test Category"), s=w568, f="Blowdown Test") -> (s? t:f=w566:string)
            n265 = local write "Test Category"(w566) -> ()
            n266 = Select(t=Page_-_Execute_State."Holding - Cal Elapse Time", s=w568, f=Page_-_Execute_State."Blowdown - Check BD Trigger") -> (s? t:f=w573:T17)
          }
          frame "Holding - Cal Elapse Time" {
            w605 = T6[] [enum."Recording Duration", enum."View Change", enum."Holding Time", enum."Press. Drop Rate"] items=["Elapse Gap Data", "Holding Time", "Recording Duration", "View Change", "Pressure stabilize timer", "Press. Drop Rate", "Init Holding Buffer"]
            n267 = Unbundle By Name(w606) -> ("Array of Elapse Time"=w607:timestamp[])
            n268 = for {
              tunnel: w607 -> [w614]
              tunnel: w605 -> [w613] mode=indexing
              shift-right: [w616] -> w604
              shift-left: w606 -> [w617]
              n269 = Index Array(array=w614, index=w613) -> (element=w612:timestamp)
              n270 = Get Date/Time In Seconds() -> (seconds since 1Jan1904=w615:timestamp)
              n271 = Subtract(x=w615, y=w612) -> (x-y=w611:dbl)
              n272 = case shown="\"Recording Duration\", \"Press. Drop Rate\"" w613 {
                selector: w613 -> [w618 w626 _ _]
                tunnel: w617 -> [w622 w630 w633 w648]
                tunnel: [w621 w629 w633 w648] -> w616
                tunnel: w611 -> [w619 w625 w634 _]
                frame "Recording Duration", "Press. Drop Rate" {
                  n273 = Unbundle By Name(w622) -> ("Result Elapse"=w623:dbl[])
                  n274 = Replace Array Subset(array=w623, new element=w619, index=w618) -> (w620:dbl[])
                  n275 = Bundle By Name(cluster=w622, "Result Elapse"=w620) -> (w621:T16)
                }
                frame "Holding Time" {
                  n276 = Unbundle By Name(w630) -> ("Result Elapse"=w627:dbl[], "Holding Started?"=w632:bool)
                  n277 = Index Array(array=w627, index=w626) -> (element=w624:dbl)
                  n278 = Select(t=w625, s=w632, f=w624) -> (s? t:f=w631:dbl)
                  n279 = Replace Array Subset(array=w627, new element=w631, index=w626) -> (w628:dbl[])
                  n280 = Bundle By Name(cluster=w630, "Result Elapse"=w628) -> (w629:T16)
                }
                frame "View Change" {
                  n281 = Unbundle By Name(w633) -> ("Default View"=w638:string, "View Change Duration"=w635:dbl)
                  n282 = local read "View"() -> (w636:string)
                  n283 = Equal?(x=w636, y=w638) -> (x = y?=w637:bool)
                  n284 = case shown="False" w637 {
                    tunnel: w635 -> [w646 _]
                    tunnel: w638 -> [w643 _]
                    tunnel: w634 -> [w642 _]
                    frame False {
                      n285 = Multiply(x=w646, y=60.0) -> (x*y=w644:dbl)
                      n286 = Greater Or Equal?(x=w642, y=w644) -> (x >= y?=w640:bool)
                      n287 = call-poly <userlib>:"Data Changed__ogtk.vi"("Boolean"=w640) -> ("Changed"=w641:bool)
                      n288 = Compound Arithmetic op=AND(w641, w640) -> (w639:bool)
                      n289 = case shown="True" w639 {
                        tunnel: w643 -> [_ w647]
                        frame False {
                        }
                        frame True {
                          n290 = property on="View" class="CmbBox"("Val(Sgnl)"=w647) -> ()  [unwired: 2 in, 2 out]
                        }
                      }
                    }
                    frame True {
                    }
                  }
                }
                frame Default {
                }
              }
            }
          }
          frame "Display Data" {
            w662 = "%H:%M:%S %B%d, %Y" ("time format string (%c)")
            w667 = 1 ("disabled index (col)")
            # "Display Pressure Data and recording Duration"
            n291 = Unbundle By Name(w665) -> ("Result Elapse"=w682:dbl[], "Run Test"=w677:bool)
            n292 = To Long Integer(number=Execute_-_Index_of_Elapse_time."Recording Duration") -> (32bit integer=w678:i32)
            n293 = Index Array(array=w682, index=w678) -> (element=w679:dbl)
            n294 = case shown="True" w677 {
              tunnel: w681 -> [w684 w688]
              tunnel: [w684 w687] -> w670
              tunnel: w679 -> [_ w686]
              frame False {
              }
              frame True {
                n295 = Format Into String(format string="%<%H:%M:%S>t", error in=w688, w686) -> (resulting string=→"Recording Duration" →"Key Value Recording Duration":string, error out=w687:errorcluster)  [unwired: 1 in]
              }
            }
            n296 = Unbundle By Name(w665) -> ("Run Pressure Data.Max Pressure"=w661:dbl, "Run Pressure Data.Min Pressure"=w658:dbl, "Run Pressure Data.Max Pressure TS"=w664:timestamp, "Run Pressure Data.Min Pressure TS"=w663:timestamp)
            n297 = Number To Fractional String(number=w661, precision (6)=i16 1) -> (F-format string=w657:string)  [unwired: 2 in]
            n298 = Number To Fractional String(number=w658, precision (6)=i16 1) -> (F-format string=w653:string)  [unwired: 2 in]
            n299 = Format Date/Time String(time format string (%c)=w662, seconds (now)=w664) -> (date/time string=w655:string)  [unwired: 1 in]
            n300 = Format Date/Time String(time format string (%c)=w662, seconds (now)=w663) -> (date/time string=w652:string)  [unwired: 1 in]
            n301 = Concatenate Strings(w657, " at " ("string"), w655) -> (w650:string)
            n302 = Concatenate Strings(w653, " at " ("string"), w652) -> (w651:string)
            n303 = property on="Table Reading" class="MCListbox (strict)"(error in=w670) -> (error out=w669:errorcluster, "ItemNames"=w672:string[][])  [unwired: 1 in, 1 out]
            n304 = Unbundle By Name(w665) -> ("Run Test"=w676:bool)
            n305 = Replace Array Subset(array=w672, new element #1=w650, index (row) #1=9 ("index (row)"), index (col) #1=w667, new element #2=w651, index (row) #2=10 ("disabled index (row)"), index (col) #2=w667) -> (w649:string[][])
            n306 = property on="Table Reading" class="MCListbox (strict)"(error in=w669, "ItemNames"=w649) -> (error out=w668:errorcluster)  [unwired: 1 in, 1 out]
            n307 = property on="Statistic" class="MCListbox (strict)"("ItemNames"=w649) -> ()  [unwired: 2 in, 2 out]
            n308 = Select(t=Page_-_Execute_State."Check pressure in range", s=w676, f=Page_-_Execute_State."Idle") -> (s? t:f=w674:T17)
          }
          frame "Check pressure in range" {
            n309 = Unbundle By Name(w706) -> ("Test Pressure Range.Maximum"=w707:dbl, "Test Pressure Range.Minimum"=w701:dbl)
            n310 = local read "Current Pressure (psi)"() -> (w697:sgl)
            n311 = In Range and Coerce(upper limit=w707, x=w697, lower limit=w701) -> (In Range?=w690:bool)  [unwired: 1 out]
            "Pressure in Range" <- w690
            n312 = call <userlib>:"Boolean Trigger__ogtk.vi"("Boolean Input"=w690) -> ("Rising Edge"=w692:bool)  [unwired: 1 in, 1 out]
            n313 = Divide(x=w697, y=w701) -> (x/y=w700:dbl)
            n314 = Multiply(x=w700, y=100.0) -> (x*y=w698:dbl)
            n315 = case shown="True" w692 {
              tunnel: w706 -> [w710 w715]
              tunnel: [w710 w714] -> w705
              frame False {
              }
              frame True {
                n316 = Unbundle By Name(w715) -> ("Array of Elapse Time"=w716:timestamp[])
                n317 = Get Date/Time In Seconds() -> (seconds since 1Jan1904=w711:timestamp)
                n318 = Replace Array Subset(array=w716, new element=w711, index=Execute_-_Index_of_Elapse_time."Init Holding Buffer") -> (w713:timestamp[])
                n319 = Bundle By Name(cluster=w715, "Array of Elapse Time"=w713) -> (w714:T16)
              }
            }
            n320 = local write "%Pressure Stabilized"(w698) -> ()
            n321 = Select(t="Pressure in range.", s=w690, f="Pressure not in range" ("String.Stabilizing status")) -> (s? t:f=w702:string)
            n322 = local write "String.Stabilizing status"(w702) -> ()
            n323 = call <userlib>:"Boolean Trigger__ogtk.vi"("Boolean Input"=w690) -> ("Falling Edge"=w693:bool)  [unwired: 1 in, 1 out]
            n324 = case shown="True" w693 {
              frame False {
              }
              frame True {
                n325 = property on="Clear Mark" class="Bool"("Val(Sgnl)"=TRUE) -> ()  [unwired: 2 in, 2 out]
              }
            }
            n326 = property on="Indicator.PressureDropRatePsi" class="DigNum (strict)"("Visible"=w690) -> ()  [unwired: 2 in, 2 out]
            n327 = property on="Bool. Press Drop In Range" class="Bool (strict)"("Visible"=w690) -> ()  [unwired: 2 in, 2 out]
            n328 = Bundle By Name(cluster=w705, "Test Pressure Range.Pressure in range?"=w690) -> (w704:T16)
            n329 = property on="Indicator.PressureDropRate%" class="DigNum (strict)"("Visible"=w690) -> ()  [unwired: 2 in, 2 out]
            n330 = Select(t=Page_-_Execute_State."Calc - Holding start Buffer Time", s=w690, f=Page_-_Execute_State."Calc. Max Min Pressure") -> (s? t:f=w694:T17)
          }
          frame "Calc - Holding start Buffer Time" {
            w724 = 60.0 ("y")
            n331 = Unbundle By Name(w735) -> ("Array of Elapse Time"=w740:timestamp[])
            n332 = Index Array(array=w740, index=Execute_-_Index_of_Elapse_time."Init Holding Buffer") -> (element=w737:timestamp)
            n333 = Get Date/Time In Seconds() -> (seconds since 1Jan1904=w738:timestamp)
            n334 = Subtract(x=w738, y=w737) -> (x-y=w723:dbl)
            n335 = Greater Or Equal?(x=w723, y=w724) -> (x >= y?=w729:bool)
            n336 = Subtract(x=w724, y=w723) -> (x-y=w718:dbl)
            n337 = Less Than 0?(x=w718) -> (x < 0?=w721:bool)
            n338 = Select(t=0.0, s=w721, f=w718) -> (s? t:f=w720:dbl)
            n339 = call <userlib>:"Boolean Trigger__ogtk.vi"("Boolean Input"=w729) -> ("Rising Edge"=w736:bool)  [unwired: 1 in, 1 out]
            n340 = Number To Decimal String(number=w720) -> (decimal integer string=w722:string)  [unwired: 1 in]
            n341 = case shown="True" w736 {
              tunnel: w735 -> [w742 w745]
              tunnel: [w742 w744] -> w734
              frame False {
              }
              frame True {
                n342 = local read "Current Pressure (psi)"() -> (w743:sgl)
                n343 = Bundle By Name(cluster=w745, "Drop Rate Param.Last Pressure (psi)"=w743) -> (w744:T16)
              }
            }
            n344 = Concatenate Strings(w722, " seconds before checking for stabilization.") -> (w717:string)
            n345 = local read "String.Stabilizing status"() -> (w733:string)
            n346 = Select(t=" Start checking for stabilization.", s=w729, f=w717) -> (s? t:f=w728:string)
            n347 = Concatenate Strings(w733, w728) -> (w727:string)
            n348 = local write "String.Stabilizing status"(w727) -> ()
            n349 = Select(t=Page_-_Execute_State."Calc. press. drop rate", s=w729, f=Page_-_Execute_State."Calc. Max Min Pressure") -> (s? t:f=w730:T17)
          }
          frame "Calc. press. drop rate" {
            n350 = Unbundle By Name(w748) -> ("Drop Rate Param.Drop Rate Calc Interval (sec)"=w759:dbl, "Current Sequence.Seq.TestPressure"=w756:string)
            n351 = Unbundle By Name(w748) -> ("Result Elapse"=w764:dbl[])
            n352 = Index Array(array=w764, index=Execute_-_Index_of_Elapse_time."Press. Drop Rate") -> (element=w762:dbl)
            n353 = Greater Or Equal?(x=w762, y=w759) -> (x >= y?=w758:bool)
            n354 = local read "Current Pressure (psi)"() -> (w750:sgl)
            n355 = Unbundle By Name(w748) -> ("Drop Rate Param"=w751:T14)
            n356 = Fract/Exp String To Number(string=w756) -> (number=w755:dbl)  [unwired: 3 in, 1 out]
            n357 = call "Calculate Pressure Drop Rate.vi"("Drop Rate Param"=w751, "Current Pressure (psi)"=w750) -> ("Drop rate within range?"=w747:bool, "Pressure drop rate/hr"=w749:dbl)  [unwired: 2 in]
            "Bool. Press Drop In Range" <- w747
            "Indicator.PressureDropRatePsi" <- w749
            n358 = case shown="False" w747 {
              tunnel: w748 -> [w770 w774]
              tunnel: [w773 w774] -> w746
              frame False {
                n359 = Unbundle By Name(w770) -> ("Array of Elapse Time"=w769:timestamp[])
                n360 = local read "Current Pressure (psi)"() -> (w771:sgl)
                n361 = Get Date/Time In Seconds() -> (seconds since 1Jan1904=w767:timestamp)
                n362 = Replace Array Subset(array=w769, new element=w767, index=Execute_-_Index_of_Elapse_time."Press. Drop Rate") -> (w766:timestamp[])
                n363 = Bundle By Name(cluster=w770, "Drop Rate Param.Block counter"=0, "Drop Rate Param.Last Pressure (psi)"=w771, "Array of Elapse Time"=w766) -> (w773:T16)
              }
              frame True {
              }
            }
            n364 = Divide(x=w749, y=w755) -> (x/y=w754:dbl)
            n365 = Multiply(x=100.0, y=w754) -> (x*y=→"Indicator.PressureDropRate%":dbl)
            n366 = Bundle By Name(cluster=w746, "Drop Rate Param.Pressure Drop Accepted?"=w747) -> (w757:T16)
            n367 = case shown="True" w758 {
              tunnel: w757 -> [w775 w784]
              tunnel: [w775 w789] -> w761
              tunnel: w747 -> [_ w781]
              frame False {
              }
              frame True {
                n368 = Unbundle By Name(w784) -> ("Drop Rate Param.Block counter"=w780:i32)
                n369 = call-poly <userlib>:"Data Changed__ogtk.vi"("Boolean"=w781) -> ("Changed"=w782:bool)
                n370 = Unbundle By Name(w784) -> ("Array of Elapse Time"=w788:timestamp[])
                n371 = Exclusive Or(1:w782, 2:w781) -> (0:w779:bool)
                n372 = Get Date/Time In Seconds() -> (seconds since 1Jan1904=w785:timestamp)
                n373 = Select(t=0, s=w779, f=w780) -> (s? t:f=w777:i32)
                n374 = Increment(x=w780) -> (x+1=w783:i32)
                n375 = Replace Array Subset(array=w788, new element=w785, index=Execute_-_Index_of_Elapse_time."Press. Drop Rate") -> (w787:timestamp[])
                n376 = Select(t=w783, s=w781, f=w777) -> (s? t:f=w776:i32)
                n377 = Bundle By Name(cluster=w784, "Array of Elapse Time"=w787, "Drop Rate Param.Block counter"=w776) -> (w789:T16)
              }
            }
          }
          frame "Calc. stabilizing elapsed time" {
            # "bypass for the sbsut1"
            n378 = Unbundle By Name(w791) -> ("Drop Rate Param.Drop Rate Calc Interval (sec)"=w795:dbl, "Drop Rate Param.Block counter"=w793:i32, "Drop Rate Param.Block interval to test"=w798:i32)
            n379 = Unbundle By Name(w791) -> ("Holding Started?"=w790:bool)
            n380 = Subtract(x=w798, y=w793) -> (x-y=w796:i32)
            n381 = Greater Or Equal?(x=w793, y=w798) -> (x >= y?=w799:bool)
            n382 = call-poly <userlib>:"Data Changed__ogtk.vi"("Boolean"=w799) -> ("Changed"=w800:bool)
            n383 = Format Into String(format string="Stabilize testing for %d blocks of %.0f seconds", w796, w795) -> (resulting string=w794:string)  [unwired: 2 in, 1 out]
            n384 = case shown="False" w790 {
              tunnel: w794 -> [w804 _]
              frame False {
                n385 = local write "String.Stabilizing status"(w804) -> ()
              }
              frame True {
              }
            }
            n386 = Compound Arithmetic op=AND(w800, w799) -> (w792:bool)
            n387 = case shown="True" w792 {
              tunnel: w803 -> [w805 w808]
              tunnel: [w805 w807] -> w802
              frame False {
              }
              frame True {
                n388 = property on="Holding Started" class="Bool (strict)"(error in=w808, "Val(Sgnl)"=TRUE ("Value (Signaling)")) -> (error out=w807:errorcluster)  [unwired: 1 in, 1 out]
              }
            }
          }
          frame "Calc. Max Min Pressure" {
            n389 = local read "Current Pressure (psi)"() -> (w814:sgl)
            n390 = Unbundle By Name(w817) -> ("Run Pressure Data.Max Pressure"=w816:dbl, "Run Pressure Data.Min Pressure"=w813:dbl)
            n391 = Greater?(x=w814, y=w816) -> (0:w818:bool)
            n392 = Less?(x=w814, y=w813) -> (x < y?=w812:bool)
            n393 = case shown="True" w818 {
              tunnel: w817 -> [w825 w829]
              tunnel: w814 -> [_ w827]
              tunnel: [w825 w828] -> w815
              frame False {
              }
              frame True {
                n394 = Get Date/Time In Seconds() -> (seconds since 1Jan1904=w826:timestamp)
                n395 = Bundle By Name(cluster=w829, "Run Pressure Data.Max Pressure"=w827, "Run Pressure Data.Max Pressure TS"=w826) -> (w828:T16)
              }
            }
            n396 = local read "Current Pressure (psi)"() -> (w811:sgl)
            n397 = case shown="True" w812 {
              tunnel: w815 -> [w820 w824]
              tunnel: w811 -> [_ w822]
              tunnel: [w820 w823] -> w810
              frame False {
              }
              frame True {
                n398 = Get Date/Time In Seconds() -> (seconds since 1Jan1904=w821:timestamp)
                n399 = Bundle By Name(cluster=w824, "Run Pressure Data.Min Pressure"=w822, "Run Pressure Data.Min Pressure TS"=w821) -> (w823:T16)
              }
            }
          }
          frame "Check Start Holding" {
          }
          frame "Blowdown - Check BD Trigger" {
            # "#CONSTANT"
            n400 = Unbundle By Name(w847) -> ("Current Sequence.Seq.TestPressure"=w846:string)
            n401 = local read "Current Pressure (psi)"() -> (w842:sgl)
            n402 = Fract/Exp String To Number(string=w846) -> (number=w845:dbl)  [unwired: 3 in, 1 out]
            n403 = Multiply(x=w845, y=0.5) -> (x*y=w843:dbl)
            n404 = local read "NumInd.2nd_pump_press"() -> (w836:sgl)
            n405 = Less Or Equal?(x=w842, y=w843) -> (x <= y?=w837:bool)
            n406 = local write "Bool.BDTrig"(w837) -> ()
            n407 = call <userlib>:"Boolean Trigger__ogtk.vi"("Boolean Input"=w837) -> ("Rising Edge"=w833:bool)  [unwired: 1 in, 1 out]
            n408 = case shown="False" w833 {
              tunnel: w847 -> [w851 w857]
              tunnel: [w850 w856] -> w841
              tunnel: w837 -> [w849 w855]
              tunnel: w836 -> [w848 w854]
              tunnel: w835 -> [w852 w853]
              tunnel: [w852 w853] -> w834
              frame False {
                n409 = local write "NumInd.BD_Pressure"(w848) -> ()
                n410 = Bundle By Name(cluster=w851, "Blowdown Param.BD Triggered"=w849, "Blowdown Param.BD Pressure"=w848) -> (w850:T16)
              }
              frame True {
                n411 = Bundle By Name(cluster=w857, "Blowdown Param.BD Triggered"=w855, "Blowdown Param.BD Pressure"=w854) -> (w856:T16)
              }
            }
            n412 = Select(t=Page_-_Execute_State."Blowdown - Mark BD", s=w837, f=Page_-_Execute_State."Polar attributes") -> (s? t:f=w838:T17)
          }
          frame "Blowdown - Mark BD" {
            # "#HASNI"
            n413 = Unbundle By Name(w859) -> ("Blowdown Param.BD Triggered"=w858:bool)
            n414 = case shown="False" w858 {
              tunnel: w859 -> [w863 w868]
              tunnel: [w863 w866] -> w860
              frame False {
              }
              frame True {
                n415 = Unbundle By Name(w868) -> ("Point Phase"=w867:dbl[], "Counter Time"=w864:dbl)
                n416 = Insert Into Array(array=w867, new element=w864) -> (w865:dbl[])  [unwired: 1 in]
                n417 = Bundle By Name(cluster=w868, "Point Phase"=w865) -> (w866:T16)
              }
            }
          }
          frame "Polar attributes" {
            w884 = 1000.0 ("y")
            # "Auto Scale"
            # "Set-up Polar attribute"
            n418 = Unbundle By Name(w879) -> ("Max Pressure"=w878:sgl, "Current Pressure"=w875:sgl)
            n419 = Greater Or Equal?(x=w878, y=w875) -> (x >= y?=w880:bool)
            n420 = Select(t=w878, s=w880, f=w875) -> (s? t:f=w874:sgl)
            n421 = Equal To 0?(x=w874) -> (x = 0?=w888:bool)
            n422 = Select(t=100.0, s=w888, f=w874) -> (s? t:f=w886:dbl)
            n423 = Multiply(x=w886, y=1.25) -> (x*y=w882:dbl)
            n424 = Divide(x=w882, y=w884) -> (x/y=w885:dbl)
            n425 = Round Toward +Infinity(x=w885) -> (ceil(x): smallest int >= x=w883:dbl)
            n426 = Multiply(x=w883, y=w884) -> (x*y=w873:dbl)
            n427 = Format Into String(format string="%.1f", w873) -> (resulting string=w871:string)  [unwired: 2 in, 1 out]
            n428 = Bundle By Name(cluster=w879, "Display Polar Scale.Max Scale label"=w871, "Max Pressure"=w874, "polar attributes.grid color"="Grid Colour", "polar attributes.plot color"="Plot Colour", "polar attributes.maximum"=w873, "polar attributes.minimum"=0.0 ("minimum"), "polar attributes.fmt and prec.format"=T21."Decimal" ("fmt and prec.format"), "Plot and scale.Size Linear plot"=u16 3, "Plot and scale.Size point plot"=u16 6) -> (w889:T16)
          }
          frame "Insert Acc Data" {
            # "Insert pressure to array of magnitude"
            n429 = Unbundle By Name(w910) -> ("Magnitude ,y"=w909:sgl[], "Current Pressure"=w908:sgl, "Time ,x"=w907:dbl[], "Result Elapse"=w906:dbl[], "Counter Time"=w904:dbl)
            n430 = To Long Integer(number=Execute_-_Index_of_Elapse_time."Elapse Gap Data") -> (32bit integer=w895:i32)
            n431 = Index Array(array=w906, index=w895) -> (element=w905:dbl)
            n432 = Add(x=w905, y=w904) -> (x+y=w900:dbl)
            n433 = Insert Into Array(array=w907, new element=w904) -> (w901:dbl[])  [unwired: 1 in]
            n434 = Insert Into Array(array=w909, new element=w908) -> (w902:sgl[])  [unwired: 1 in]
            n435 = Bundle By Name(cluster=w910, "Magnitude ,y"=w902, "Time ,x"=w901, "Counter Time"=w900) -> (w903:T16)
          }
          frame "Convert Time To Phase" {
            # "Convert time to phase"
            n436 = Unbundle By Name(w925) -> ("Magnitude ,y"=w918:sgl[], "Time ,x"=w924:dbl[], "Plot length scale"=w912:dbl, "Point Phase"=w914:dbl[])
            n437 = Multiply(x=w924, y=w912) -> (x*y=w919:dbl[])
            n438 = for {
              shift-right: [w932] -> w920
              shift-left: w921 -> [w932]
              tunnel: w919 -> [w927] mode=indexing
              tunnel: w918 -> [w929] mode=indexing
              tunnel: [w930] -> w915 mode=indexing
              tunnel: [w927] -> w916
              tunnel: w912 -> [w926]
              tunnel: [w926] -> w911
              n439 = To Double Precision Float(number=w929) -> (double precision float=w928:dbl)
              n440 = Bundle By Name(cluster=cluster{"magnitude":dbl, "phase":dbl} {"magnitude"=0.0, "phase"=0.0} ("data array [mag, phase (deg)]"), "magnitude"=w928, "phase"=w927) -> (w930:cluster{"magnitude":dbl, "phase":dbl})
            }
            n441 = call "Execute Search To Mark.vi"("Plot length scale"=w911, "Point Phase"=w914, "Data [magnitude,Phase]In"=w915) -> ("Data [magnitude,Phase] Out"=w913:cluster{"magnitude 2":dbl, "phase":dbl}[])  [unwired: 8 in]
            n442 = Bundle By Name(cluster=w925, "data array [mag, phase (deg)]"=w915, "Max Phase"=w916, "Marking Data"=w913) -> (w922:T16)
          }
          frame "Get Plot length" {
            n443 = Unbundle By Name(w951) -> ("Plot length (min)"=w950:dbl, "Plot length scale"=w949:dbl, "Max Phase"=w948:dbl)
            n444 = call "Get plot length.vi"("Max phase"=w948, "Plot length scale"=w949, "Plot length (min)"=w950) -> ("New plot length scale"=w946:dbl, "New plot length"=w935:dbl)
            n445 = Multiply(x=w935, y=60.0) -> (x*y=w941:dbl)
            n446 = To Long Integer(number=w935) -> (32bit integer=w943:i32)
            n447 = Multiply(x=w941, y=dbl[] [0.0, 0.041666666666666664, 0.08333333333333333, 0.125, 0.16666666666666666, 0.20833333333333334, 0.25, 0.2916666666666667, 0.3333333333333333, 0.375, 0.4166666666666667, 0.4583333333333333, 0.5, 0.5416666666666666, 0.5833333333333334, 0.625, 0.6666666666666666, 0.7083333333333334, 0.75, 0.7916666666666666, 0.8333333333333334, 0.875, 0.9166666666666666, 0.9583333333333334, 1.0] ("Array 2")) -> (x*y=w940:dbl[])
            n448 = Format Into String(format string="%d", w943) -> (resulting string=w942:string)  [unwired: 2 in, 1 out]
            n449 = for {
              tunnel: w940 -> [w955] mode=indexing
              tunnel: [w953] -> w934 mode=indexing
              shift-right: [w952] -> w936
              shift-left: w937 -> [w952]
              n450 = Number To Fractional String(number=w955, precision (6)=i16 1) -> (F-format string=w953:string)  [unwired: 2 in]
            }
            n451 = Bundle By Name(cluster=w951, "Display Polar Scale.Time Scale Label"=w942, "Plot length (min)"=w935, "Plot length scale"=w946, "axis labels"=w934) -> (w947:T16)
          }
          frame "Polar linear Plot" {
            # "plot polar data"
            n452 = Unbundle By Name(w970) -> ("Plot and scale"=w966:T29, "data array [mag, phase (deg)]"=w967:cluster{"magnitude":dbl, "phase":dbl}[], "polar attributes"=w969:T30, "axis labels"=w964:string[])
            n453 = Unbundle By Name(w966) -> ("Plot Scale"=w956:dbl, "Size Linear plot"=w957:u16)
            n454 = property on="Polar Plot" class="Pict"(error in=w968) -> (error out=w961:errorcluster, "Draw Area Size"=w960:T31)  [unwired: 1 in, 1 out]
            n455 = Bundle By Name(cluster=T22 {"polar attributes"={"maximum"=0.0, "minimum"=0.0, "clip to min"=FALSE, "log?(F)"=FALSE, "grid color"=6710886, "plot color"=16711680, "fmt and prec"={"format"=enum."Decimal", "precision"=0}, "visible section"=8}, "data array [mag, phase (deg)]"=[], "font"={"desired font(Application) "=enum."Application Font", "[user-specified font] "={"Font Name:"="", "Size"=0, "Strikeout?"=FALSE, "Italic?"=FALSE, "Underline?"=FALSE, "Outline?"=FALSE, "Shadow?"=FALSE, "Bold?"=FALSE}}, "Scale Polar plot"=0.2, "Size"=1} ("Polar Properties"), "Scale Polar plot"=w956, "Size"=w957, "data array [mag, phase (deg)]"=w967, "polar attributes"=w969) -> (w959:T22)
            n456 = call "Polar Plot-Linear.vi"("axis labels"=w964, "error in"=w961, "dimensions (w,h)"=w960, "Polar Properties"=w959) -> ("error Out"=w965:errorcluster, "picture out"=w962:picture)  [unwired: 6 in]
            n457 = Bundle By Name(cluster=w970, "Polar Picture"=w962) -> (w963:T16)
          }
          frame "Polar Point" {
            # "plot polar data"
            n458 = Unbundle By Name(w977) -> ("Polar Picture"=w974:picture, "Plot and scale"=w987:T29, "marking plot colour"=w988:u32, "Marking Data"=w989:cluster{"magnitude 2":dbl, "phase":dbl}[], "polar attributes"=w991:T30, "axis labels"=w986:string[])
            n459 = Bundle By Name(cluster=w991, "plot color"=w988) -> (w978:T30)
            n460 = Unbundle By Name(w987) -> ("Plot Scale"=w980:dbl, "Size point plot"=w981:u16)
            n461 = property on="Polar Plot" class="Pict"(error in=w990) -> (error out=w985:errorcluster, "Draw Area Size"=w984:T31)  [unwired: 1 in, 1 out]
            n462 = Bundle By Name(cluster=T22 {"polar attributes"={"maximum"=0.0, "minimum"=0.0, "clip to min"=FALSE, "log?(F)"=FALSE, "grid color"=6710886, "plot color"=16711680, "fmt and prec"={"format"=enum."Decimal", "precision"=0}, "visible section"=8}, "data array [mag, phase (deg)]"=[], "font"={"desired font(Application) "=enum."Application Font", "[user-specified font] "={"Font Name:"="", "Size"=0, "Strikeout?"=FALSE, "Italic?"=FALSE, "Underline?"=FALSE, "Outline?"=FALSE, "Shadow?"=FALSE, "Bold?"=FALSE}}, "Scale Polar plot"=0.2, "Size"=1} ("Polar Properties"), "Scale Polar plot"=w980, "Size"=w981, "data array [mag, phase (deg)]"=w989, "polar attributes"=w978) -> (w983:T22)
            n463 = call "Polar Plot-Point.vi"("axis labels"=w986, "error in"=w985, "dimensions (w,h)"=w984, "Polar Properties"=w983, "picture In"=w974) -> ("error Out"=w979:errorcluster, "picture out"=w973:picture)  [unwired: 5 in]
            n464 = Bundle By Name(cluster=w977, "Polar Picture"=w973) -> (w975:T16)
          }
          frame "Display Label" {
            n465 = Unbundle By Name(w997) -> ("Display Polar Scale.Max Scale label"=w995:string, "Display Polar Scale.Time Scale Label"=w996:string, "Polar Picture"=w994:picture)
            n466 = call <vilib>:"Space Constant.vi"() -> ("String"=w1005:string)
            n467 = Concatenate Strings("1 rev = " ("text"), w996, w1005, "Minute" ("string")) -> (w1007:string)
            n468 = call <vilib>:"Space Constant.vi"() -> ("String"=w1001:string)
            n469 = Concatenate Strings("Max Scale  = " ("text"), w995, w1001, "psi" ("string")) -> (w998:string)
            n470 = call <vilib>:"Draw Text at Point.vi"("text"=w1007, "origin"=cluster{"x":i16, "y":i16} {"x"=722, "y"=35}, "picture"=w994) -> ("new picture"=w1003:picture)  [unwired: 7 in, 1 out]
            n471 = call <vilib>:"Draw Text at Point.vi"("text"=w998, "origin"=cluster{"x":i16, "y":i16} {"x"=722, "y"=15}, "picture"=w1003) -> ("new picture"=→"Polar Plot":picture)  [unwired: 7 in, 1 out]
          }
          frame "Plot linear Graph" {
            # "Display sensor ata on linear graph"
            n472 = Unbundle By Name(w1019) -> ("Time ,x"=w1021:dbl[], "Magnitude ,y"=w1020:sgl[])
            n473 = Bundle By Name(cluster=cluster{"Time ,x":dbl[], "Magnitude ,y":sgl[]} {"Time ,x"=[], "Magnitude ,y"=[]}, "Time ,x"=w1021, "Magnitude ,y"=w1020) -> (→"Linear Graph":cluster{"Time ,x":dbl[], "Magnitude ,y":sgl[]})
            n474 = Unbundle By Name(w1019) -> ("Point Phase"=w1018:dbl[])
            n475 = Array Size(array=w1018) -> (size(s)=w1017:i32)
            n476 = Not Equal?(x=w1017, y=1) -> (x != y?=w1015:bool)
            n477 = Select(t=Page_-_Execute_State."Idle", s=w1015, f=Page_-_Execute_State."Update Table Data") -> (s? t:f=w1013:T17)
          }
          frame "Update Table Data" {
          }
          frame "Display Holding Time" {
            n478 = Unbundle By Name(w1045) -> ("Result Elapse"=w1043:dbl[], "Remaining Holding Time"=w1039:dbl, "Target Holding Time"=w1037:dbl)
            n479 = To Long Integer(number=Execute_-_Index_of_Elapse_time."Holding Time") -> (32bit integer=w1041:i32)
            n480 = Index Array(array=w1043, index=w1041) -> (element=w1040:dbl)
            n481 = Subtract(x=w1039, y=w1040) -> (x-y=w1031:dbl)
            "Hold Time Remainder" <- w1031
            n482 = Subtract(x=w1037, y=w1031) -> (x-y=w1038:dbl)
            n483 = Divide(x=w1038, y=w1037) -> (x/y=w1036:dbl)
            n484 = Less Than 0?(x=w1031) -> (x < 0?=w1033:bool)
            n485 = Multiply(x=w1036, y=100.0) -> (x*y=→"% Test Completed":dbl)
            n486 = Select(t=0.0, s=w1033, f=w1031) -> (s? t:f=w1030:dbl)
            n487 = Format Into String(format string="%<%H:%M:%S>t", error in=w1049, w1030) -> (resulting string=→"Remaining Hold Time":string, error out=w1048:errorcluster)  [unwired: 1 in]
            n488 = Less Or Equal To 0?(x=w1031) -> (x <= 0?=w1046:bool)
            n489 = case shown="True" w1046 {
              tunnel: w1048 -> [w1053 w1062]
              tunnel: [w1053 w1054] -> w1047
              tunnel: w1045 -> [w1052 w1065]
              tunnel: [w1052 w1064] -> w1044
              frame False {
              }
              frame True {
                n490 = property on="End Mark" class="Bool (strict)"(error in=w1062, "Val(Sgnl)"=TRUE) -> (error out=w1066:errorcluster)  [unwired: 1 in, 1 out]
                n491 = Get Date/Time In Seconds() -> (seconds since 1Jan1904=w1058:timestamp)
                n492 = property on="Table Reading" class="MCListbox (strict)"(error in=w1066) -> ("ItemNames"=w1059:string[][])  [unwired: 1 in, 2 out]
                n493 = Format Date/Time String(time format string (%c)="%H:%M:%S %B%d, %y", seconds (now)=w1058) -> (date/time string=w1061:string)  [unwired: 1 in]
                n494 = Bundle By Name(cluster=w1065, "Start Mark"=FALSE) -> (w1064:T16)
                n495 = Replace Array Subset(array=w1059, new element=w1061, index (row)=1 ("disabled index (row)"), index (col)=1 ("disabled index (col)")) -> (w1060:string[][])
                n496 = property on="Table Reading" class="MCListbox (strict)"("ItemNames"=w1060) -> (error out=w1054:errorcluster)  [unwired: 2 in, 1 out]
              }
            }
          }
          frame "Display Result Test" {
            w1074 = 1 ("index (row)")
            n497 = Unbundle By Name(w1087) -> ("Start Holding Pressure (psi)"=w1081:dbl, "Remaining Holding Time"=w1086:dbl)
            n498 = Format Into String(format string="%<%H:%M:%S>t", error in=w1095, w1086) -> (resulting string=w1075:string, error out=w1082:errorcluster)  [unwired: 1 in]
            "Recorded Holding Time" <- w1075
            n499 = property on="Current Pressure (psi)" class="DigNum (strict)"(error in=w1082) -> (error out=w1094:errorcluster, "Value"=w1080:sgl)  [unwired: 1 in, 1 out]
            n500 = Subtract(x=w1080, y=w1081) -> (x-y=w1090:dbl)
            n501 = Absolute Value(x=w1090) -> (abs(x)=w1088:dbl)
            n502 = Divide(x=w1088, y=w1081) -> (x/y=w1069:dbl)
            n503 = local read "Recording Duration"() -> (w1072:string)
            n504 = Not A Number/Path/Refnum?(number/path/refnum=w1069) -> (NaN/Path/Refnum?=w1071:bool)
            n505 = Select(t=0.0, s=w1071, f=w1069) -> (s? t:f=w1068:dbl)
            n506 = Multiply(x=w1068, y=100.0) -> (x*y=w1089:dbl)
            n507 = Format Into String(format string="%.1f psi(%.1f %%)", w1088, w1089) -> (resulting string=w1076:string)  [unwired: 2 in, 1 out]
            "Different in Holding Pressure,psi(%)" <- w1076
            n508 = property on="Table Reading" class="MCListbox (strict)"(error in=w1094) -> (error out=w1085:errorcluster, "ItemNames"=w1083:string[][])  [unwired: 1 in, 1 out]
            n509 = Replace Array Subset(array=w1083, new element #1=w1076, index (row) #1=5 ("index (row)"), index (col) #1=w1074, new element #2=w1075, index (row) #2=2 ("index (row)"), index (col) #2=w1074, new element #3=w1072, index (row) #3=8 ("disabled index (row)"), index (col) #3=w1074) -> (w1084:string[][])
            n510 = property on="Table Reading" class="MCListbox (strict)"(error in=w1085, "ItemNames"=w1084) -> (error out=w1079:errorcluster)  [unwired: 1 in, 1 out]
          }
          frame "Finish Test" {
            n511 = Unbundle By Name(w1101) -> ("Sequence Data"=w1104:T13[], "Sequence Number"=w1102:i32)
            n512 = Index Array(array=w1104, index=w1102) -> (element=w1106:T13)
            n513 = Bundle By Name(cluster=w1106, "Seq.Status"=u32 6618880) -> (w1103:T13)
            n514 = Replace Array Subset(array=w1104, new element=w1103, index=w1102) -> (w1099:T13[])
            n515 = Bundle By Name(cluster=w1101, "Sequence Data"=w1099) -> (w1100:T16)
            n516 = local write "Sequence List"(w1099) -> ()
          }
          frame "Save  Data" {
            w1114 = "Passed" ("Test Status Ind")
            n517 = Unbundle By Name(w1137) -> ("Data to Execute.Transaction Info.Transaction Number"=w1109:string)
            n518 = call "FGV - Data Path.vi"("FGV State"=State_-_FGV."Read", "Error In"=w1145) -> ("Error Out"=w1140:errorcluster, "Path Out"=w1127:path)  [unwired: 8 in]
            n519 = Build Path(base path=w1127, name or relative path=path "Results") -> (appended path=w1136:path)
            n520 = Build Path(base path=w1136, name or relative path=w1109) -> (appended path=w1134:path)
            n521 = local read "SequenceNoFolder"() -> (w1133:string)
            n522 = Build Path(base path=w1134, name or relative path=w1133) -> (appended path=w1126:path)
            n523 = invoke on="Polar Plot" class="Pict" method="Get Image"(error in=w1140) -> (error out=w1139:errorcluster, "image data"=w1138:T32)  [unwired: 5 in, 4 out]
            n524 = Concatenate Strings("Polar" ("string"), ".jpeg") -> (w1142:string)
            n525 = Build Path(base path=w1126, name or relative path=w1142) -> (appended path=w1144:path)
            n526 = call <vilib>:"Write JPEG File.vi"("quality (80)"=100, "error in (no error)"=w1139, "image data"=w1138, "path to JPEG file"=w1144) -> ("error out"=w1125:errorcluster)  [unwired: 6 in, 1 out]
            n527 = invoke on="Linear Graph" class="XYGraph (strict)" method="Get Image"(error in=w1125) -> (error out=w1124:errorcluster, "image data"=w1123:T32)  [unwired: 5 in, 4 out]
            n528 = Concatenate Strings("Linear" ("string"), ".jpeg") -> (w1130:string)
            n529 = Build Path(base path=w1126, name or relative path=w1130) -> (appended path=w1128:path)
            n530 = call <vilib>:"Write JPEG File.vi"("quality (80)"=100, "error in (no error)"=w1124, "image data"=w1123, "path to JPEG file"=w1128) -> ("error out"=w1110:errorcluster)  [unwired: 6 in, 1 out]
            n531 = property on="Table Reading" class="MCListbox (strict)"() -> ("ItemNames"=w1122:string[][])  [unwired: 2 in, 2 out]
            n532 = local read "SequenceNoFolder"() -> (w1118:string)
            n533 = local write "Test Status Ind"(w1114) -> ()
            n534 = Replace Array Subset(array=w1122, new element=w1114, index (row)=7, index (col)=1 ("disabled index (col)")) -> (w1120:string[][])
            n535 = property on="Table Reading" class="MCListbox (strict)"("ItemNames"=w1120) -> ()  [unwired: 2 in, 2 out]
            n536 = Index Array(array=w1120, index (col)=1 ("disabled index (col)")) -> (element=w1119:string[])  [unwired: 1 in]
            n537 = Bundle By Name(cluster=T23 {"Execute Data"=[], "Sequence no"=""} ("Data To Report"), "Execute Data"=w1119, "Sequence no"=w1118) -> (w1121:T23)
            n538 = call "eFGV - Data to Report.vi"("Action"=State_-_eFGV."Write", "Error In"=w1110, "Data To Report"=w1121) -> ("Error Out"=w1111:errorcluster)  [unwired: 7 in, 1 out]
          }
          frame "Get Next Sequence" {
            n539 = Unbundle By Name(w1157) -> ("Sequence Number"=w1153:i32, "Sequence Data"=w1154:T13[])
            n540 = Array Size(array=w1154) -> (size(s)=w1152:i32)
            n541 = Decrement(x=w1152) -> (x-1=w1151:i32)
            n542 = Less?(x=w1153, y=w1151) -> (x < y?=w1150:bool)
            n543 = case shown="True" w1150 {
              tunnel: w1157 -> [w1165 w1171]
              tunnel: [Page_-_Execute_State."Idle" Page_-_Execute_State."Get Current Sequence"] -> w1156
              tunnel: [w1164 w1169] -> w1155
              tunnel: w1153 -> [_ w1167]
              frame False {
                n544 = Bundle By Name(cluster=w1165, "Sequence Number"=0, "All Sequence Done"=TRUE) -> (w1164:T16)
                n545 = call "Gen - Popup Single Button (Auto Close).vi"("Message in"="All test sequence are done", "Header"="TEST SEQUENCE") -> ()  [unwired: 8 in, 2 out]
              }
              frame True {
                n546 = Increment(x=w1167) -> (x+1=w1168:i32)
                n547 = Bundle By Name(cluster=w1171, "Sequence Number"=w1168, "Sequence Started"=FALSE) -> (w1169:T16)
              }
            }
          }
          frame "Create Report" {
            n548 = call <vilib>:"Create Report.vi"("report type"=Report_Type."Excel", "error in (no error)"=w1176) -> ("report out"=w1173:refnum<class "NI_report.lvclass">, "error out"=w1175:errorcluster)  [unwired: 12 in]
            n549 = Bundle By Name(cluster=w1179, "report out"=w1173) -> (w1174:T16)
          }
          frame "Fillup Report" {
            n550 = Unbundle By Name(w1186) -> ("report out"=w1185:refnum<class "NI_report.lvclass">)
            n551 = call-poly <vilib>:"Append Report Text.vi"("report in"=w1185, "MS Office parameters"=T26 {"position (excel)"={"row"=0, "column"=0}, "name (excel)"="", "bookmark (word)"=""}, "text"="", "error in (no error)"=w1187) -> ("report out"=w1184:refnum<class "NI_report.lvclass">, "error out"=w1183:errorcluster)  [unwired: 8 in, 2 out]
            n552 = call-dynamic "Dispose Report.vi"("report in"=w1184, "error in (no error)"=w1183) -> ("error out"=w1182:errorcluster)  [unwired: 13 in]
          }
          frame "Process" {
          }
          frame "Update Info - Transaction" {
            n553 = Unbundle By Name(w1205) -> ("Data to Execute.Transaction Info"=w1204:T8)
            n554 = Unbundle By Name(w1204) -> ("Quantity"=w1203:u16, "Customer"=w1202:u32, "Customer Description"=w1200:string, "Project"=w1199:string, "Sales Order"=w1198:u32, "Material Description"=w1196:string, "Rework"=w1195:bool, "NCR No."=w1194:string, "BOM Rev."=w1193:dbl)  [unwired: 4 out]
            n555 = Number To Decimal String(number=w1202) -> (decimal integer string=w1201:string)  [unwired: 1 in]
            n556 = Number To Decimal String(number=w1198) -> (decimal integer string=w1197:string)  [unwired: 1 in]
            n557 = local write "Quantity"(w1203) -> ()
            n558 = local write "Customer"(w1201) -> ()
            n559 = local write "Customer Description"(w1200) -> ()
            n560 = local write "Project"(w1199) -> ()
            n561 = local write "Sale Order"(w1197) -> ()
            n562 = local write "Material Description"(w1196) -> ()
            n563 = local write "Rework"(w1195) -> ()
            n564 = local write "NCR No."(w1194) -> ()
            n565 = local write "BOM Rev."(w1193) -> ()
          }
          frame "Update Info - Product" {
            n566 = Unbundle By Name(w1216) -> ("Data to Execute.Product Info.Product Category"=w1215:string, "Data to Execute.Product Info.Procedure No./Ref."=w1214:string, "Data to Execute.Product Info.Test System"=w1208:string, "Data to Execute.Product Info.Test System Description"=w1213:string, "Data to Execute.Product Info.Working Pressure"=w1212:string, "Data to Execute.Product Info.Rev."=w1211:string, "Data to Execute.Product Info.PSL"=w1210:string)
            n567 = local write "Product Category"(w1215) -> ()
            n568 = local write "Procedure No./Ref."(w1214) -> ()
            n569 = local write "Test System"(w1208) -> ()
            n570 = local write "Test System Description"(w1213) -> ()
            n571 = local write "Working Pressure"(w1212) -> ()
            n572 = local write "Rev."(w1211) -> ()
            n573 = local write "PSL"(w1210) -> ()
            n574 = local write "Test System"(w1208) -> ()
          }
          frame "Update Info - Additional Refs" {
            n575 = Unbundle By Name(w1222) -> ("Data to Execute.Misc - Additional Refs"=w1219:string[][])
            n576 = property on="Table.Procedure No./Ref." class="MCListbox (strict)"(error in=w1221, "ItemNames"=w1219) -> (error out=w1220:errorcluster)  [unwired: 1 in, 1 out]
          }
          frame "Update Info - Sensors" {
            n577 = Unbundle By Name(w1227) -> ("Data to Execute.Misc - Sensors"=w1224:string[][])
            n578 = property on="Table.Sensor" class="MCListbox (strict)"(error in=w1226, "ItemNames"=w1224) -> (error out=w1225:errorcluster)  [unwired: 1 in, 1 out]
          }
          frame "Update Info - Tools" {
            n579 = Unbundle By Name(w1232) -> ("Data to Execute.Misc - Tools"=w1229:string[][])
            n580 = property on="Table.Tool" class="MCListbox (strict)"(error in=w1231, "ItemNames"=w1229) -> (error out=w1230:errorcluster)  [unwired: 1 in, 1 out]
          }
          frame "Update Info - Acceptance Criteria" {
            n581 = Unbundle By Name(w1249) -> ("Data to Execute.Acceptance Criteria Info.Max Start Hold Pressure"=w1239:dbl, "Data to Execute.Acceptance Criteria Info.Permitted Hold Pressure Drop"=w1248:dbl, "Data to Execute.Acceptance Criteria Info.Enum.Max Start Hold Pressure"=w1240:enum16{"%", "psi"}, "Data to Execute.Acceptance Criteria Info.Enum.Permitted Hold Pressure Drop"=w1238:enum16{"%", "psi"}, "Data to Execute.Acceptance Criteria Info.Pressure stabilize wait time"=w1234:dbl, "Data to Execute.Acceptance Criteria Info.Enum.Pressure stabilize wait time"=w1236:enum16{"seconds", "minutes"})
            n582 = local write "Pressure stabilize wait time"(w1234) -> ()
            n583 = local write "Enum.Pressure stabilize wait time"(w1236) -> ()
            n584 = Format Into String(w1240) -> (resulting string=w1247:string)  [unwired: 3 in, 1 out]
            n585 = Format Into String(w1238) -> (resulting string=w1244:string)  [unwired: 3 in, 1 out]
            n586 = local write "Max Start Holding Pressure"(w1239) -> ()
            n587 = local write "Permitted Holding Pressure Drop"(w1248) -> ()
            n588 = case shown="\"seconds\", Default" w1236 {
              tunnel: [1.0 60.0] -> w1235
              frame "seconds", Default {
              }
              frame "minutes" {
              }
            }
            n589 = Multiply(x=w1234, y=w1235) -> (x*y=w1233:dbl)
            n590 = Concatenate Strings(w1247, " on top of the test pressure" ("string")) -> (w1243:string)
            n591 = Concatenate Strings(w1244, " per hour (vs. start holding pressure)" ("string")) -> (w1242:string)
            n592 = local write "% Test Pressure"(w1243) -> ()
            n593 = local write "% Permitted Holding Pressure"(w1242) -> ()
            n594 = Bundle By Name(cluster=w1249, "Drop Rate Param.Drop Rate Calc Interval (sec)"=w1233) -> (w1237:T16)
          }
          frame "Update Info - Execution" {
            n595 = Unbundle By Name(w1261) -> ("Data to Execute.Execution Info.Auto Set Marker"=w1256:bool, "Data to Execute.Execution Info.Auto Stop Test"=w1260:bool)
            n596 = local write "Auto Set Marker"(w1256) -> ()
            n597 = Select(t=T27."Disabled and Grayed Out" ("Disabled"), s=w1256, f=T27."Enabled") -> (s? t:f=w1253:T27)
            n598 = local write "Auto Stop Test"(w1260) -> ()
            n599 = property on="Start Mark" class="Bool (strict)"(error in=w1258, "DisabledEnum"=w1253) -> (error out=w1257:errorcluster)  [unwired: 1 in, 1 out]
          }
          frame "Update Info - Results" {
            n600 = Unbundle By Name(w1265) -> ("Data to Execute.Results Info.ListBox.Output Set"=w1264:string, "Data to Execute.Results Info.Output Set Description"=w1263:string)
            n601 = local write "ListBox.Output Set"(w1264) -> ()
            n602 = local write "Output Set Company"(w1263) -> ()
          }
          frame "Update Info - Notes" {
            n603 = Unbundle By Name(w1268) -> ("Data to Execute.Notes"=w1267:string)
            n604 = local write "Notes"(w1267) -> ()
          }
          frame "Close" {
            n605 = Unbundle By Name(w1272) -> ("Event Ref"=w1271:refnum<event-registration>)
            n606 = Unregister For Events(event registration refnum=w1271, error in=w1276) -> (error out=w1275:errorcluster)
          }
        }
      }
      frame Error {
        n607 = call <vilib>:"Clear Errors.vi"("error in (no error)"=w1280) -> ("error out"=w1283:errorcluster)  [unwired: 5 in, 1 out]
        n608 = call "Gen - Get Application Kind.vi"("Error In"=w1283) -> ("Error Out"=w1279:errorcluster, "Application:Kind"=w1282:T33)  [unwired: 9 in]
        n609 = Format Into String(error in=w1279, w1277) -> (resulting string=w1278:string)  [unwired: 2 in, 1 out]
        n610 = case shown="\"Development System\"" w1282 {
          tunnel: [w1287 w1292 w1296] -> w1281
          tunnel: w1280 -> [w1287 w1289 w1294]
          tunnel: w1278 -> [_ w1288 _]
          frame "invalid app kind", Default {
          }
          frame "Run Time System" {
            n611 = control-ref of="This VI"() -> (w1290:refnum<vi>)
            n612 = call "eFGV - Generated Error.vi"("eFGV States"=State_-_eFGV."Write", "Error In"=w1289, "State"=w1288, "This VI"=w1290) -> ("Error Out"=w1292:errorcluster)  [unwired: 6 in, 1 out]
          }
          frame "Development System" {
            n613 = call <vilib>:"Simple Error Handler.vi"("error in (no error)"=w1294) -> ("error?"=w1293:bool, "error out"=w1295:errorcluster)  [unwired: 4 in, 3 out]
            n614 = case shown="False" w1293 {
              tunnel: [w1297 w1299] -> w1296
              tunnel: w1295 -> [w1297 w1298]
              frame False {
              }
              frame True {
                n615 = call <vilib>:"Clear Errors.vi"("error in (no error)"=w1298) -> ("error out"=w1299:errorcluster)  [unwired: 5 in, 1 out]
              }
            }
          }
        }
      }
    }
  }
